vi "UHR-Fleezers Control (fpga) - 11.5_testing.vi"() -> ()   [LabVIEW 2012]
doc: "UHR-Fleezers Instrument Control Code (fpga)"
uses:
  Downloads/HandshakingLV2011/Handshaking/FPGAHandShakeState.ctl
  <vilib>/Platform/TimedLoop/XDataNode/timing_clust.ctl
  <vilib>/Platform/TimedLoop/XDataNode/nitl_modes.ctl
  <vilib>/Platform/TimedLoop/XDataNode/wakeup.ctl
  <vilib>/rvi/eio/common/nirviEmuTemplateMethod_errors.vi
  <vilib>/rvi/Emulation/niFpgaSctlEmulationGetInTimedLoop.vi
  <vilib>/rvi/DataTransferAndStorage/Container/Common/niFpgaContainerGetUniqueNameForEmu.vi
  <vilib>/rvi/FIFO/Fifo_Resource/nirvififoEmulationSetSize.vi
  <vilib>/rvi/Emulation/niFpgaSctlEmulationFifoFullMgr.vi
  <vilib>/rvi/errors/niFpgaSetErrorForExecOnDevCompSimple.vi
  <vilib>/rvi/eio/common/nirviEmuReportErrorAndStop.vi
  <vilib>/rvi/interface/RandomDataEmulation/nirviRandomDataFPGAFIFO.vi
  <vilib>/rvi/interface/RandomDataEmulation/niFpgaRandomDataHandleErrors.vi
  <vilib>/rvi/Emulation/niFpgaSctlEmulationGlobalWrite.vi
  <vilib>/rvi/Emulation/niFpgaSctlEmulationRegisterWithScheduler.vi
  <vilib>/rvi/Emulation/niFpgaSctlEmulationScheduler.vi
  <vilib>/rvi/DataTransferAndStorage/Container/Common/niFpgaContainerExecOnDevCompGetState.vi
  <vilib>/rvi/Memory/Memory_Emulation/niFpgaMemoryEmulationCacheClearOnFirstRun.vi
  <vilib>/rvi/Memory/Memory_Emulation/nirvimemoryEmulationManagerCache_MakeExclusive.vi
  <vilib>/rvi/Memory/Memory_Emulation/niFpgaMemoryEmulationValidateCache.vi
  <vilib>/rvi/Memory/Memory_Emulation/nirvimemoryEmulationManagerCache_ReleaseExclusive.vi
  <vilib>/rvi/Memory/Memory_Emulation/nirvimemoryEmulationManagerCache_InsertValue.vi
  <vilib>/Utility/error.llb/Clear Errors.vi
  <vilib>/rvi/Memory/Memory_Emulation/nirvimemoryEmulationManagerCache_GetValue.vi
  <vilib>/rvi/Memory/Memory_Emulation/nirvimemoryEmulationManagerCache_SetValue.vi
  <vilib>/rvi/Emulation/niFpgaSctlEmulationResourceMgr.vi
  <vilib>/Platform/TimedLoop/XDataNode/XDataNode.xnode
  <vilib>/eio/EIOMethodNode/EIOMethodNode.xnode
  <vilib>/eio/EIONode/EIONode.xnode
  <vilib>/rvi/DataTransferAndStorage/Container/XNode/niFpgaContainer.xnode
  <vilib>/rvi/FIFO/Fifo_Resource/nirvififoEmulationRead.vi
  <vilib>/rvi/interface/RandomDataEmulation/nirviRandomDataFpgaReadWriteTemplate.vi
  <vilib>/rvi/Memory/Memory_Emulation/niFpgaMemoryEmulationRefIn.vi
  <vilib>/rvi/FIFO/Fifo_Resource/nirvififoEmulationWrite.vi
  <vilib>/addons/control/pid/fpga.llb/XNode/niFpgaPID.xnode
  <vilib>/Platform/TimedLoop/XDataNode/XDNodeRunTimeDep.lvlib
panel:
  in  "N trap osc periods":i16
  in  "Trap osc period (pts)":i16
  in  "Initiate trap osc":bool
  in  "Osc trap 2":bool
  in  "Data":i32
  in  "Address 2":u32
  in  "Ready Write":bool
  in  "Tab Control":T1(tab)=enum."Force FB"
  in  "Set 3":bool
  in  "Set 2":bool=TRUE
  in  "Set 1":bool=TRUE
  in  "Trap Pos to FIFO":bool
  in  "N of AI1 Int Acq Sets":i16=2 min=1 max=3 step=1
  out "AI Late Counter":u8
  in  "ai count":u16=400
  in  "+ phase":bool
  in  "Phase count adjustment":i16
  out "Relative phase":i16
  in  "AI to FIFO":bool
  out "BD1 Frequency Out 1":u64
  out "BD1 Frequency Out 2":u64
  out "Trap Pos FIFO Timeout":u16
  out "Trap AI FIFO Timeout":u16
  in  "Trap FIFO Set Timeout":i32
  in  "Tab Control 2":T2(tab)
  in  "RD":bool
  in  "FB1 output high":i16=3000
  in  "FB1 output low":i16
  in  "D1":i16
  in  "I1":i16=5
  in  "P1":i16=10
  in  "Swap F1 and F2":bool
  in  "Cont. Scan":bool
  in  "Abort scan":bool
  in  "Cycles per step":u64
  in  "Scan BD":bool
  in  "Number of scans":u16
  in  "Scan steps":u64
  in  "Scan freq.  increment":i64
  out "Scanning":bool
  in  "Start scan":bool
  in  "OSK Bd 1":bool
  in  "Reset Bd 1":bool
  in  "PMODE":bool
  in  "Direct RF Box \nCommunication":bool
  in  "Data BD 2":u8 format="%08b"
  in  "Data BD 1":u8 format="%08b"
  in  "Address":u8 format="%02x"
  in  "Update Data":bool
  in  "FPGA Controls\n RF Box":bool
  in  "Number Interlace Cycles":u8=2 min=1 max=3
  in  "Interlace Off Parameters":u8=1 min=1 max=3
  in  "Interlace ON/OFF":bool
  out "DIO Relative phase":i16
  in  "Phase count adjustment (DIO)":i16
  in  "+ phase (DIO)":bool
  out "DIO Late Counter":u8
  in  "DIO count 1 (ticks)":u16=400
  in  "DIO count 2 (ticks)":u16=400
  in  "DIO count 3 (ticks)":u16=400
  out "AI2 Y Sum Set 2":i16
  out "AI2 Y Sum Set 1":i16
  in  "FB Setpoint Set 1":i16 min=0 step=1
  in  "FB Reset Set 1":bool
  in  "FB On/Off Set 1":bool
  in  "FB Reset Set 2":bool
  in  "FB On/Off Set 2":bool
  in  "FB Setpoint Set 2":i16 min=0 step=1
  out "Scan I":u64
  in  "Amp switch delay":u8=5
  in  "XY phase ext loop method":bool
  in  "BD 2 Amplitude 1":u16
  in  "BD 1 Amplitude 1":u16
  in  "BD 2 Frequency 1":u64
  in  "BD 1 Frequency 1":u64
  in  "BD 2 Amplitude 2":u16
  in  "BD 1 Amplitude 2":u16
  in  "BD 2 Frequency 2":u64
  in  "BD 1 Frequency 2":u64
  in  "BD 2 Amplitude 3":u16
  in  "BD 1 Amplitude 3":u16
  in  "BD 2 Frequency 3":u64
  in  "BD 1 Frequency 3":u64
  in  "BD 1 Delay (ticks)":u8
  in  "BD 2 Delay (Ticks)":u8 caption="Count(Ticks)"
  in  "Next trap write delay (ticks)":u8 caption="Count(Ticks)"
  in  "Amp switch delay 2":u8=5
  in  "BD 2 Delay (Ticks) 2":u8 caption="Count(Ticks)"
  in  "BD 1 Delay (ticks) 2":u8
  in  "FB2 output high":fxp<+/-,16,1>=0.999969482421875
  in  "FB2 output low":fxp<+/-,16,1>=-1.0
  in  "P2":fxp<+/-,16,8> format="%.11g"
  in  "I2":fxp<+/-,16,8>=10.0 format="%.11g"
  in  "D2":fxp<+/-,16,8> format="%.11g"
  in  "Negate Diff?":bool
  in  "Diff FB Measurement?":bool
  in  "FB Trig Integrate":u32=1
  out "TTrig?":bool
  in  "TTrig Negate Pos":bool=TRUE
  out "Trap Pos FB Int Signal":fxp<+/-,24,9> format="%.18g"
  out "Trap Pos FB Int-Norm Signal":fxp<+/-,16,1> format="%.16g"
  in  "FPGA TTrig Thresh":i64
  in  "FPGA Trap Trig":bool
  out "Trap Pos FB Action":i64
  in  "Trap Pos. FB Offset Factor":i64
  in  "Trap Pos. FB Mult Factor":i64=2
  in  "Trap Pos. FB Reset":bool
  in  "Trap Pos FB Monitor T1 or T2":bool
  in  "AI1 X Scale":u16
  in  "Trap Pos FB Int Count":u16=100
  in  "Trap Pos FB Negate Action":bool
  out "AI1 X Set 2":fxp<+/-,16,1>
  out "AI1 X Set 1":fxp<+/-,16,1>
  in  "Trap Pos. FB SP":fxp<+/-,16,1>
  in  "Force feedback":bool
  out "TTrig Sig":i64
  out "TTrig Fin Thresh":i64
  in  "1D or 2D Scan?":bool
  in  "Abort scan (MCL)":bool
  in  "MCL Scan Axis":bool
  in  "Cont. Scan (MCL)":bool
  out "Scan I (MCL)":u64
  in  "Number of scans (MCL)":u16
  out "Scanning MCL":bool
  in  "Scan steps (MCL)":u64
  in  "Cycles per step (MCL)":u64
  in  "Scan freq.  increment (MCL)":i16
  in  "Start scan (MCL)":bool
  in  "AO2":i16
  in  "AO1":i16
  out "MCL Late Counter":u8
  in  "MCL count":u32=800
  out "MCL Relative Phase":i16
  in  "Phase count adjustment (MCL)":i16
  in  "+ phase (MCL)":bool
  out "APD3 out state":bool
  in  "APD Gate Operating Mode":u8 max=2 step=1
  in  "Invert APD Gate":bool
  in  "APD Gate OFF Count":u16=100
  in  "APD Gate ON Count":u16=300
  out "APD 1 Gate Late Counter":u8
  out "APD 1 Gate Relative Phase":i16
  in  "Phase count adjustment (APD 1 Gate)":i16
  in  "+ phase (APD 1 Gate)":bool
  out "APD 2 Counts 0":u32
  out "APD 2 Counts 1":u32
  out "APD 1 Counts 0":u32
  out "APD 1 Counts 1":u32
  out "APD1 out state":bool
  in  "APD AO scale factor":i16=1
  in  "APD to FIFO":bool
  in  "APD Acq Rate Count":u32=20000000
  out "APD Acq Late Counter":u8
  out "APD Acq Relative Phase":i16
  in  "Phase Count Adjustment (APD Acq)":i16
  in  "+ phase (APD Acq)":bool
  in  "Phase count adjustment (APD 2 Gate)":i16
  out "APD 2 Gate Late Counter":u8
  out "APD 2 Gate Relative Phase":i16
  in  "+ phase (APD 2 Gate)":bool
  out "APD2 out state":bool
  out "APD 3 Counts 0":u32
  out "APD 3 Counts 1":u32
  out "APD 3 Gate Late Counter":u8
  in  "Phase count adjustment (APD 3 Gate)":i16
  out "APD 3 Gate Relative Phase":i16
  in  "+ phase (APD 3 Gate)":bool
  in  "D3":i16
  in  "I3":i16=5
  in  "P3":i16=10
  in  "Green Filter Flipper":bool
  in  "Green FB Count":u16=1200
  out "Green Late Counter":u8
  out "Green FB Relative Phase":i16
  in  "Phase count adjustment (Green FB)":i16=10
  in  "+ phase (Green FB)":bool
  out "Green FB Sum":i16
  in  "Green int current ON count adj":u16=150
  in  "Current Out":u16=30000
  in  "Green FB On/Off":bool
  in  "Green FB Setpoint":i16=250 min=0 step=1
  in  "Green FB Reset":bool
  in  "Operating Mode 2":u8=2 max=2 step=1
  in  "Invert GI 2":bool
  in  "Green interlace OFF count 2":u16=900
  in  "Green interlace ON count 2":u16=300
  out "GI Late Counter 2":u8
  out "GI Relative phase 2":i16
  in  "Phase count adjustment (GI) 2":i16=20
  in  "+ phase (GI) 2":bool
  in  "Green interlace OFF count":u16=100
  out "GI Relative phase":i16
  in  "Phase count adjustment (GI)":i16
  in  "+ phase (GI)":bool
  in  "Green interlace ON count":u16=300
  out "GI Late Counter":u8
  in  "Invert GI":bool
  in  "Operating Mode":u8 max=2 step=1
  in  "+ phase (RI)":bool
  out "RI Relative phase":i16
  out "RI Late Counter":u8
  in  "Red interlace ON count":u16=300
  in  "Red interlace OFF count":u16=100
  in  "Invert RI":bool
  in  "Red Laser Operating Mode":u8 max=2 step=1
  in  "Phase count adjustment (RI)":i16
  out "Red FB Intensity":i16
  in  "RI Current Out":u16=30000
  in  "Red FB On/Off":bool
  in  "D4":i16
  in  "I4":i16=5
  in  "P4":i16=10
  in  "Red FB Setpoint":i16=250 min=0 step=1
  in  "Red FB Reset":bool
  in  "RI Operating Mode 2":u8=2 max=2 step=1
  in  "Invert RI 2":bool
  in  "Phase count adjustment (BI AO)":i16=20
  in  "Blue current ON count adj (AO)":u16=150
  in  "BI Current Out":i16=30000
  in  "Blue FB On/Off":bool
  in  "D5":i16
  in  "I5":i16=5
  in  "P5":i16=10
  in  "Blue FB Setpoint":i16=250 min=0 step=1
  in  "Blue FB Reset":bool
  in  "BI Operating Mode (AO)":u8=2 max=2 step=1
  in  "Invert BI (AO)":bool
  in  "Blue OFF count (AO)":u16=900
  in  "Blue ON count (AO)":u16=300
  out "BI Late Counter (AO)":u8
  out "BI Relative phase (AO)":i16
  in  "+ phase (BI AO)":bool
  in  "Phase count adjustment (BI D)":i16
  in  "Blue Laser Operating Mode (D)":u8 max=2 step=1
  in  "Invert BI (D)":bool
  in  "Blue interlace OFF count (D)":u16=100
  in  "Blue interlace ON count (D)":u16=300
  out "Blue Late Counter (D)":u8
  out "BI Relative phase (D)":i16
  in  "+ phase (BI D)":bool
  out "Blue Intensity":i16
  # "Only one of these can be on\nat a time:"
  # "Raster Scan AOD"
  # "1 (X)"
  # "2 (Y)"
  # "IR Intensity Feedback (RF BD 1)"
  # "FB Gains Set 1"
  # "FB output range 1"
  # "False is usual, True is external loop method"
  # "Parameters if using the external RF switching loop"
  # "Parameters if using the usual internal RF switching method"
  # "FB Triggering Excitation Laser"
  # "Trap Pos. FB Gains"
  # "Trap Pos. FB Range"
  # "AO1 (Y)"
  # "2D"
  # "1D"
  # "AO2 (X)"
  # "APD AO for aligning"
  # "Detection Loop"
  # "Green fluorescent laser digital gate interlacing loop"
  # "0 Forced ON\n1 Forced OFF\n2 Interlacing"
  # "Green FB Gains"
  # "Red fluorescent laser digital gate interlacing loop"
  # "Detection Loop"
  # "0 Forced ON\n1 Forced OFF\n2 Interlacing"
  # "Analog/FB Control Loop\n(Disabled)"
  # "Digital Control Loop"
  # "Blue laser intensity reading"
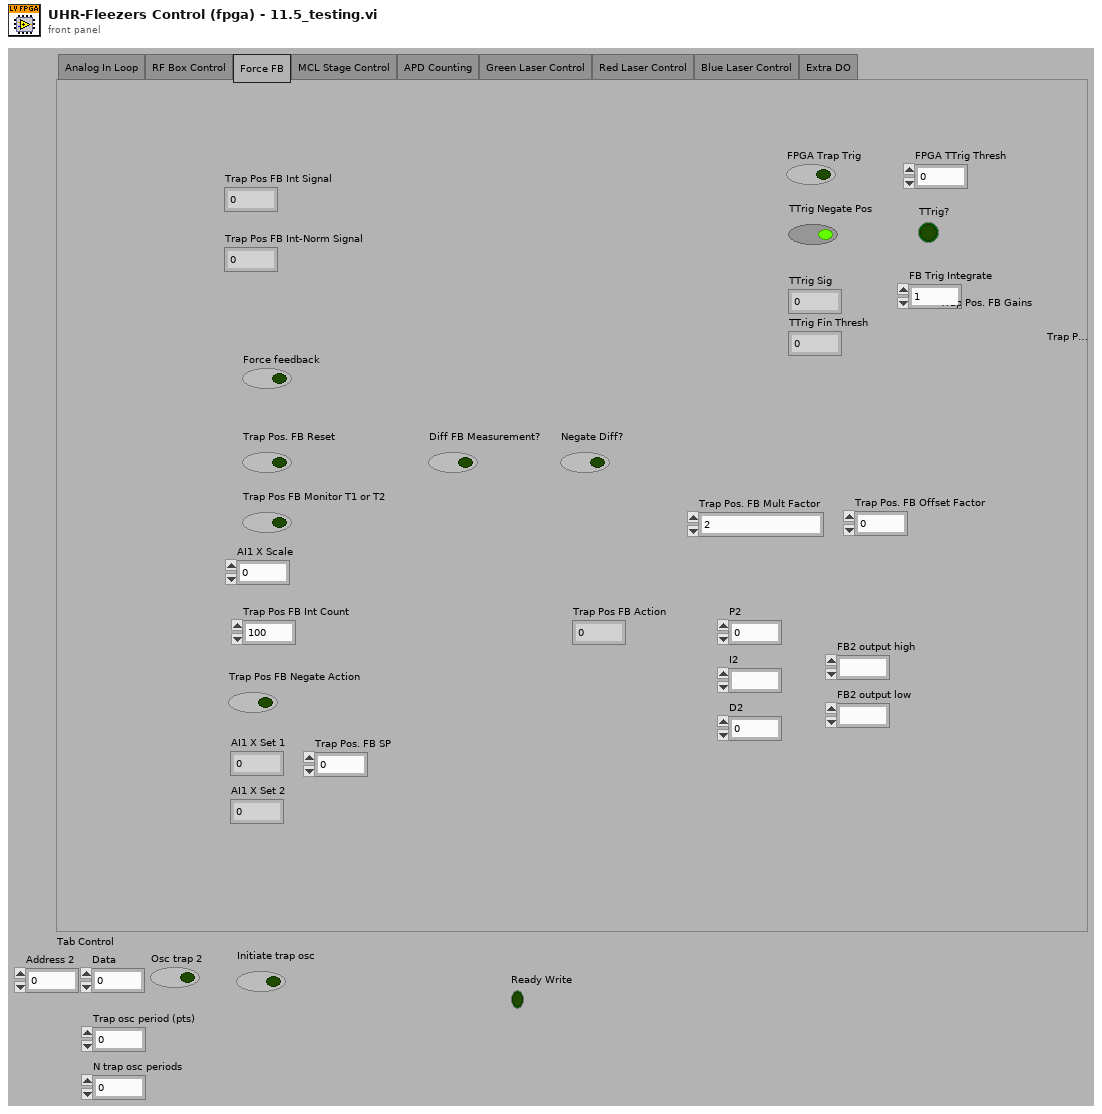
[diagram p1: front panel]
types:
  T1 = enum32{"Analog In Loop", "RF Box Control", "Force FB", "MCL Stage Control", "APD Counting", "Green Laser Control", "Red Laser Control", "Blue Laser Control", "Extra DO"}
  T2 = enum32{"Controls", "Interlacing Frequency and Amplitude Values"}
  T3 = typedef "FPGAHandShakeState.ctl" = enum16{"Wait Ready", "ReadWrite", "UnSet Ready"}
  T4 = typedef "XDNodeRunTimeDep.lvlib/timing_clust.ctl" = cluster{"Expected End [f-1]":u64, "Actual End [f-1]":u64, "Finished Late? [f-1]":bool, "Expected End [i-1]":u64, "Actual End [i-1]":u64, "Finished Late? [i-1]":bool, "Expected Start [i]":u64, "Actual Start [i]":u64, "Expected Start [f]":u64, "Actual Start [f]":u64, "Source Name":string, "Structure Name":string, "Period":i64, "Deadline":i64, "Offset":i64, "Start":i64, "Priority":i32, "Timeout":i32, "Mode":T5, "Wakeup Reason":T6, "Error":errorcluster, "Source Type":string, "Secondary Source Type":string, "Global End Time":u64, "Global Start Time":u64, "Frame Duration":u64, "Iteration Duration":u64, "Assigned CPU":i32, "I/O Scan Engine Mode":u32}
  T5 = typedef "XDNodeRunTimeDep.lvlib/nitl_modes.ctl" = enum32{"No Change", "Process missed periods, maintain original phase", "Discard missed periods, maintain original phase", "Process missed periods, ignore original phase", "Discard missed periods, ignore original phase"}
  T6 = typedef "XDNodeRunTimeDep.lvlib/wakeup.ctl" = enum32{"Normal", "Aborted", "Asynchronous wakeup", "Timing source error", "Timed loop error", "Timeout"}
  T7 = cluster{"proportional gain (Kc)":i16, "integral gain (Kc*Ts/Ti)":i16, "derivative gain (Kc*Td/Ts)":i16}
  T8 = cluster{"FB1 output high":i16, "FB1 output low":i16}
  T9 = cluster{"P2":fxp<+/-,16,8>, "I2":fxp<+/-,16,8>, "D2":fxp<+/-,16,8>}
  T10 = cluster{"FB2 output high":fxp<+/-,16,1>, "FB2 output low":fxp<+/-,16,1>}
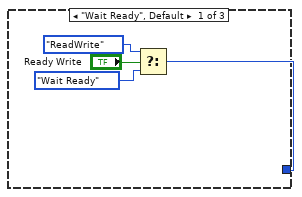
[diagram p2: hidden frame]
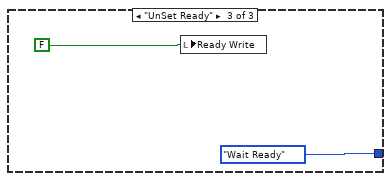
[diagram p3: hidden frame]
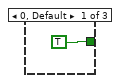
[diagram p5: hidden frame]
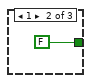
[diagram p6: hidden frame]
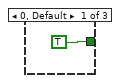
[diagram p7: hidden frame]
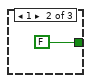
[diagram p8: hidden frame]
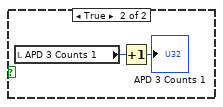
[diagram p9: hidden frame]
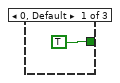
[diagram p10: hidden frame]
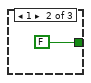
[diagram p11: hidden frame]
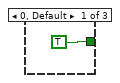
[diagram p12: hidden frame]
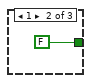
[diagram p13: hidden frame]
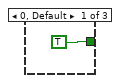
[diagram p14: hidden frame]
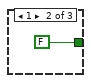
[diagram p15: hidden frame]
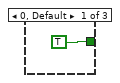
[diagram p16: hidden frame]
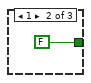
[diagram p17: hidden frame]
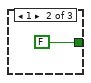
[diagram p20: hidden frame]
diagram:
  w4 = u16 0
  w6 = FALSE
  w3 = FALSE
  # "timing array current index"
  # "timing array"
  # "timing counter (phase adjusted here)"
  # "late counter"
  n1 = while "External XY RF switching timing loop" {
    stop <- FALSE stop-if-true
    # "This loop is stalled until the RF FIFO get a value, which only happens if we are using the external loop RF switching method. With this method we gain additional delay time (because \nwe allow the rest of the main RF loop to procede while this loop waits to send the switch signals - a form of parallelism). Probably this is always the method to use. Helps to simplify \nthe main RF code. If it works reliably, could take out the redundant code in the main RF loop to save space and simplify."
    n2 = xnode "FIFO Read"("Timeout"=-1) -> ("Element"=w16:bool)  [unwired: 1 in, 2 out]
    n3 = flat-sequence "BD 1 (X)" {
      tunnel: w16 -> [w25]
      tunnel: [w25] -> w15
      tunnel: w15 -> [w27]
      tunnel: "Amp switch delay 2" -> [w28]
      frame #0 {
        n4 = call "Wait9"("Count(Ticks)"="BD 1 Delay (ticks) 2") -> ()  [unwired: 1 out]
      }
      frame #1 {
        # "switch frequency"
        n5 = xnode "FPGA I/O Node"("Connector1/DIO36"=w27) -> ()  [unwired: 1 in, 1 out]
      }
      frame #2 {
        # "~5 ticks is usual"
        n6 = call "Wait10"("Count(Ticks)"=w28) -> ()  [unwired: 1 out]
      }
      frame #3 {
        # "this switches amplitude"
        # "switch amplitude"
        # "send udclk high"
        n7 = xnode "FPGA I/O Node"("Connector1/DIO30"=TRUE ("Connector1/DIO15")) -> ()  [unwired: 1 in, 1 out]
      }
      frame #4 {
        # "reset to be ready for next\ncycle"
        # "send udclk low"
        n8 = xnode "FPGA I/O Node"("Connector1/DIO30"=FALSE ("Connector1/DIO15")) -> ()  [unwired: 1 in, 1 out]
      }
    }
    n9 = flat-sequence "BD 2 (Y)" {
      tunnel: w16 -> [w19]
      tunnel: [w19] -> w14
      tunnel: w14 -> [w21]
      tunnel: "Amp switch delay 2" -> [w22]
      frame #0 {
        n10 = call "Wait11"("Count(Ticks)"="BD 2 Delay (Ticks) 2") -> ()  [unwired: 1 out]
      }
      frame #1 {
        # "switch frequency"
        n11 = xnode "FPGA I/O Node"("Connector1/DIO37"=w21) -> ()  [unwired: 1 in, 1 out]
      }
      frame #2 {
        # "~5 ticks is usual"
        n12 = call "Wait12"("Count(Ticks)"=w22) -> ()  [unwired: 1 out]
      }
      frame #3 {
        # "this switches amplitude"
        # "switch amplitude"
        # "send udclk high"
        n13 = xnode "FPGA I/O Node"("Connector1/DIO29"=TRUE ("Connector1/DIO15")) -> ()  [unwired: 1 in, 1 out]
      }
      frame #4 {
        # "reset to be ready for next\ncycle"
        # "send udclk low"
        n14 = xnode "FPGA I/O Node"("Connector1/DIO29"=FALSE ("Connector1/DIO15")) -> ()  [unwired: 1 in, 1 out]
      }
    }
  }
  n15 = flat-sequence "FPGA initialization to do before running any of the loops" {
    tunnel: [u16 0 ("DIO count 3 (ticks)")] -> w2
    tunnel: [w32] -> _
    frame #0 {
      w31 = FALSE ("Enable")
      # "BD 2 (Y)"
      # "BD 1 (X)"
      # "Start up expansion chassis early\nto avoid delays later"
      # "This pin controls udclk on the RF boards.\nWhen initially configuring the boards, this pin needs to be\nconfigured as a high impedance input.  Later it will be switched\nto an output."
      # "Initial setting of DIO data and \naddress to low (before reset).  \nThis needs to happen before the other\ncontrol method loops execute."
      n16 = xnode "FPGA I/O Node"("Chassis2/Mod4/AO0"=u16 0) -> ("Chassis2/Mod1/AI0"=w32:i16)  [unwired: 2 in, 2 out]
      n17 = xnode "FPGA I/O Method Node"("Enable"=w31) -> ()  [unwired: 1 in, 1 out]
      n18 = xnode "FPGA I/O Method Node"("Enable"=w31) -> ()  [unwired: 1 in, 1 out]
      n19 = xnode "FPGA I/O Node"("Connector1/DIO0"=FALSE, "Connector1/DIO1"=FALSE, "Connector1/DIO2"=FALSE, "Connector1/DIO3"=FALSE, "Connector1/DIO4"=FALSE, "Connector1/DIO5"=FALSE, "Connector1/DIO6"=FALSE, "Connector1/DIO7"=FALSE, "Connector1/DIO8"=FALSE, "Connector1/DIO9"=FALSE, "Connector1/DIO10"=FALSE, "Connector1/DIO11"=FALSE, "Connector1/DIO12"=FALSE, "Connector1/DIO13"=FALSE, "Connector1/DIO15"=FALSE, "Connector1/DIO20"=FALSE, "Connector1/DIO21"=FALSE, "Connector1/DIO22"=FALSE, "Connector1/DIO23"=FALSE, "Connector1/DIO24"=FALSE, "Connector1/DIO25"=FALSE, "Connector1/DIO26"=FALSE, "Connector1/DIO27"=FALSE, "Connector1/DIO14"=FALSE) -> ()  [unwired: 24 in, 24 out]
    }
  }
  n20 = local read "AO1"() -> (w11:i16)
  n21 = local read "AO2"() -> (w10:i16)
  n22 = node-c288() -> (w9:T4)  [unwired: 1 in]
  n23 = timed-loop "RF box board DIO control: control bits" {
    timing: w9 -> [_]
    timing-out: [_] -> w8
    tunnel: [w61] -> _
    tunnel: w2 -> [w61]
    stop <- FALSE stop-if-true
    n24 = xnode "FPGA I/O Node"("Connector1/DIO16"="RD", "Connector1/DIO17"="PMODE", "Connector1/DIO18"="OSK Bd 1", "Connector1/DIO19"="Reset Bd 1", "Connector0/DIO3"="Green Filter Flipper") -> ()  [unwired: 5 in, 5 out]
  }
  n25 = while "RF box board DIO control: parallel communication" {
    shift-right: [w74] -> _
    shift-left: w2 -> [w73]
    shift-right: [w72] -> _
    shift-left: FALSE ("Swap F1 and F2") -> [w71]
    stop <- FALSE stop-if-true
    n26 = flat-sequence {
      tunnel: w71 -> [w78]
      tunnel: w73 -> [w76]
      tunnel: [w78] -> w70
      tunnel: [w77] -> w69
      tunnel: [w76] -> w68
      tunnel: [w84] -> w74
      tunnel: [w83] -> w72
      tunnel: w70 -> [w82]
      tunnel: w69 -> [w80]
      tunnel: w68 -> [w79]
      frame #0 {
        n27 = call "Loop Timer"("Count(Ticks)"=w76) -> ("Tick Count(Ticks)"=w77:u16)
      }
      frame #1 {
        n28 = flat-sequence {
          tunnel: ["FPGA Controls\n RF Box"] -> w81
          tunnel: w82 -> [w85]
          tunnel: [w139] -> w84
          tunnel: [w152] -> w83
          tunnel: w81 -> [w151]
          tunnel: w80 -> [w145]
          tunnel: w79 -> [w142]
          frame #0 {
            n29 = case shown="True" "FPGA Controls\n RF Box" {
              tunnel: w85 -> [_ w87]
              frame False {
              }
              frame True {
                n30 = flat-sequence {
                  tunnel: w87 -> [w97]
                  frame #0 {
                    n31 = First Call?() -> (First Call?: T/F=w88:bool)
                    n32 = case shown="True" w88 {
                      frame False {
                      }
                      frame True {
                        # "BD 2"
                        # "BD 1"
                        # "If first time data updated, be sure to set WR high and UDCLK low\nbefore setting data and address bits."
                        n33 = xnode "FPGA I/O Method Node"("Enable"=TRUE) -> ("FPGA I/O Out"=w90:refnum<k21>)  [unwired: 1 in]
                        n34 = xnode "FPGA I/O Method Node"("Enable"=TRUE) -> ("FPGA I/O Out"=w93:refnum<k21>)  [unwired: 1 in]
                        n35 = xnode "FPGA I/O Node"("Connector1/DIO15"=TRUE) -> ()  [unwired: 1 in, 1 out]
                        n36 = xnode "FPGA I/O Node"("I/O Item"=FALSE ("Connector1/DIO30"), "FPGA I/O In"=w90) -> ()  [unwired: 1 out]
                        n37 = xnode "FPGA I/O Node"("I/O Item"=FALSE ("Connector1/DIO30"), "FPGA I/O In"=w93) -> ()  [unwired: 1 out]
                      }
                    }
                  }
                  frame #1 {
                    n38 = case shown="True" "XY phase ext loop method" {
                      tunnel: w97 -> [w99 w111]
                      frame False {
                        # "Usual operation"
                        n39 = flat-sequence "BD 1 (X)" {
                          tunnel: w99 -> [w106]
                          tunnel: "Amp switch delay" -> [w107]
                          frame #0 {
                            n40 = call "Wait6"("Count(Ticks)"="BD 1 Delay (ticks)") -> ()  [unwired: 1 out]
                          }
                          frame #1 {
                            # "switch frequency"
                            n41 = xnode "FPGA I/O Node"("Connector1/DIO36"=w106) -> ()  [unwired: 1 in, 1 out]
                          }
                          frame #2 {
                            # "~5 ticks is usual"
                            n42 = call "Wait4"("Count(Ticks)"=w107) -> ()  [unwired: 1 out]
                          }
                          frame #3 {
                            # "this switches amplitude"
                            # "switch amplitude"
                            # "send udclk high"
                            n43 = xnode "FPGA I/O Node"("Connector1/DIO30"=TRUE ("Connector1/DIO15")) -> ()  [unwired: 1 in, 1 out]
                          }
                          frame #4 {
                            # "reset to be ready for next\ncycle"
                            # "send udclk low"
                            n44 = xnode "FPGA I/O Node"("Connector1/DIO30"=FALSE ("Connector1/DIO15")) -> ()  [unwired: 1 in, 1 out]
                          }
                        }
                        n45 = flat-sequence "BD 2 (Y)" {
                          tunnel: w99 -> [w101]
                          tunnel: "Amp switch delay" -> [w102]
                          frame #0 {
                            n46 = call "Wait7"("Count(Ticks)"="BD 2 Delay (Ticks)") -> ()  [unwired: 1 out]
                          }
                          frame #1 {
                            # "switch frequency"
                            n47 = xnode "FPGA I/O Node"("Connector1/DIO37"=w101) -> ()  [unwired: 1 in, 1 out]
                          }
                          frame #2 {
                            # "~5 ticks is usual"
                            n48 = call "Wait5"("Count(Ticks)"=w102) -> ()  [unwired: 1 out]
                          }
                          frame #3 {
                            # "this switches amplitude"
                            # "switch amplitude"
                            # "send udclk high"
                            n49 = xnode "FPGA I/O Node"("Connector1/DIO29"=TRUE ("Connector1/DIO15")) -> ()  [unwired: 1 in, 1 out]
                          }
                          frame #4 {
                            # "reset to be ready for next\ncycle"
                            # "send udclk low"
                            n50 = xnode "FPGA I/O Node"("Connector1/DIO29"=FALSE ("Connector1/DIO15")) -> ()  [unwired: 1 in, 1 out]
                          }
                        }
                      }
                      frame True {
                        # "Operation when you need a long delay for either X or Y to synchonize AOD light out phase (> ~100 ticks)."
                        # "Trigger the external loop by sending the boolean FSK value through a FIFO"
                        n51 = xnode "FIFO Write"("Element"=w111, "Timeout"=-1) -> ()  [unwired: 1 in, 2 out]
                      }
                    }
                  }
                }
              }
            }
          }
          frame #1 {
            # "This is the prior cycle's on time"
            # "increment timing\nindex, reset to 0 if \nend of matrix"
            # "Reset to begginning (1) when number of cycles reached."
            # "timing index"
            # "build byte stacks for writing data\n(must correspond to addresses array constant)"
            # "Timing housekeeping"
            # "Adjust phase if late\n(maintains constant phase relationship between cycles)"
            n52 = Bundle("FB1 output high"="FB1 output high", "FB1 output low"="FB1 output low") -> (w112:T8)  [unwired: 1 in]
            n53 = Bundle("P1"="P1", "I1"="I1", "D1"="D1") -> (w113:cluster{"P1":i16, "I1":i16, "D1":i16})  [unwired: 1 in]
            n54 = feedback #1(u8 0 ("t")) -> (w148:u8)
            n55 = Increment(x=w148) -> (x+1=w192:u8)
            n56 = Increment(x="Number Interlace Cycles") -> (x+1=w187:u8)
            n57 = Equal?(x=w192, y=w187) -> (x = y?=w194:bool)
            n58 = Select(t=u8 1, s=w194, f=w192) -> (s? t:f=w147:u8)
            n59 = feedback-in #1(w147) -> ()
            n60 = Increment(x=w147) -> (x+1=w189:u8)
            n61 = Equal?(x=w189, y=w187) -> (x = y?=w190:bool)
            n62 = Select(t=u8 1, s=w190, f=w189) -> (s? t:f=w186:u8)
            n63 = Select(t=w186, s="Interlace ON/OFF", f="Interlace Off Parameters") -> (s? t:f=w170:u8)
            n64 = case shown="2" w170 {
              tunnel: [w271 "BD 1 Frequency 2" "BD 1 Frequency 3"] -> w182
              tunnel: [w270 "BD 2 Frequency 2" "BD 2 Frequency 3"] -> w171
              tunnel: ["BD 2 Amplitude 1" "BD 2 Amplitude 2" "BD 2 Amplitude 3"] -> w127
              tunnel: [w259 w435 "BD 1 Amplitude 3"] -> w130
              tunnel: w113 -> [w233 w432 _]
              tunnel: w112 -> [w234 w431 _]
              frame 1, Default {
                w250 = fxp<+/-,24,9> 0.0 ("AI1 X Set 2")
                w243 = u16 0
                w266 = u64 0 ("f")
                # "This signal integration happens no matter what\nso that correct setpoints can be chosen before \nturning on the FB."
                # "Trap 1"
                n65 = local read "AI1 X Set 2"() -> (w246:fxp<+/-,16,1>)
                n66 = local read "AI1 X Set 1"() -> (w247:fxp<+/-,16,1>)
                n67 = local read "Scanning"() -> (w272:bool)
                n68 = Or(x=w272, y="Start scan") -> (x .or. y?=w264:bool)
                n69 = case shown="False" "Diff FB Measurement?" {
                  tunnel: w246 -> [w280 w289]
                  tunnel: w247 -> [w279 w290]
                  tunnel: [w277 w281] -> w248
                  frame False {
                    n70 = Select(t=w279, s="Trap Pos FB Monitor T1 or T2", f=w280) -> (s? t:f=w277:fxp<+/-,16,1>)
                  }
                  frame True {
                    n71 = Subtract(x=w290, y=w289) -> (x-y=w282:fxp<+/-,17,2>)
                    n72 = Not(x="Negate Diff?") -> (.not. x?=w288:bool)
                    n73 = Boolean To (0,1)(Boolean="Negate Diff?") -> (0, 1=w286:i16)
                    n74 = Boolean To (0,1)(Boolean=w288) -> (0, 1=w287:i16)
                    n75 = Negate(x=w286) -> (-x=w285:i16)
                    n76 = Add(x=w285, y=w287) -> (x+y=w283:i16)
                    n77 = Multiply(x=w283, y=w282) -> (x*y=w281:fxp<+/-,32,17>)
                  }
                }
                n78 = Not(x="Abort scan") -> (.not. x?=w262:bool)
                n79 = And(x=w262, y=w264) -> (x .and. y?=w261:bool)
                n80 = case "For raster scanning" shown="True" w261 {
                  tunnel: [u64 0 w416] -> w267
                  tunnel: "Start scan" -> [_ w401]
                  frame False {
                    n81 = local write "Scanning"(FALSE ("scanning")) -> ()
                  }
                  frame True {
                    w385 = i64 0
                    w384 = u64 0
                    # "scan incr."
                    # "freq. incr. mult."
                    # "count steps"
                    # "count number of cycles"
                    n82 = feedback #2(w384) -> (w413:u64)
                    n83 = Select(t=w384, s=w401, f=w413) -> (s? t:f=w415:u64)
                    n84 = Increment(x=w415) -> (x+1=w412:u64)
                    n85 = Greater?(x="Cycles per step", y=w412) -> (0:w394:bool)
                    n86 = Select(t=w412, s=w394, f=w384) -> (s? t:f=w411:u64)
                    n87 = feedback-in #2(w411) -> ()
                    n88 = feedback #3(w384) -> (w410:u64)
                    n89 = Select(t=w384, s=w401, f=w410) -> (s? t:f=w405:u64)
                    n90 = Increment(x=w405) -> (x+1=w409:u64)
                    n91 = Add(x="Scan steps", y="Scan steps") -> (x+y=w408:u64)
                    n92 = Select(t=w405, s=w394, f=w409) -> (s? t:f=w389:u64)
                    n93 = Greater?(x=w408, y=w389) -> (0:w388:bool)
                    n94 = Select(t=w389, s=w388, f=w384) -> (s? t:f=w406:u64)
                    n95 = feedback-in #3(w406) -> ()
                    n96 = Equal?(x="Scan steps", y=w389) -> (x = y?=w393:bool)
                    n97 = Greater?(x="Scan steps", y=w405) -> (0:w404:bool)
                    n98 = feedback #4(w385) -> (w407:i64)
                    n99 = Select(t=w385, s=w401, f=w407) -> (s? t:f=w391:i64)
                    n100 = Increment(x=w391) -> (x+1=w403:i64)
                    n101 = Decrement(x=w391) -> (x-1=w402:i64)
                    n102 = Select(t=w403, s=w404, f=w402) -> (s? t:f=w392:i64)
                    n103 = Select(t=w391, s=w393, f=w392) -> (s? t:f=w390:i64)
                    n104 = Select(t=w391, s=w394, f=w390) -> (s? t:f=w386:i64)
                    n105 = Select(t=w386, s=w388, f=w385) -> (s? t:f=w387:i64)
                    n106 = feedback-in #4(w387) -> ()
                    n107 = feedback #5(w384) -> (w400:u64)
                    n108 = Select(t=w384, s=w401, f=w400) -> (s? t:f=w396:u64)
                    n109 = Increment(x=w396) -> (x+1=w397:u64)
                    n110 = Select(t=w396, s=w388, f=w397) -> (s? t:f=w395:u64)
                    n111 = Greater?(x="Number of scans", y=w395) -> (0:w381:bool)
                    n112 = Multiply(x="Scan freq.  increment", y=w391) -> (x*y=w416:i64)
                    n113 = Select(t=TRUE, s="Cont. Scan", f=w381) -> (s? t:f=w380:bool)
                    "Scanning" <- w380
                    n114 = Select(t=w395, s=w380, f=w384) -> (s? t:f=w398:u64)
                    n115 = feedback-in #5(w398) -> ()
                    n116 = Increment(x=w395) -> (x+1=→"Scan I":u64)
                  }
                }
                n117 = feedback #6(w243) -> (w242:u16)
                n118 = Increment(x=w242) -> (x+1=w244:u16)
                n119 = Greater Or Equal?(x=w244, y="Trap Pos FB Int Count") -> (x >= y?=w235:bool)
                n120 = Select(t=w243, s=w235, f=w244) -> (s? t:f=w245:u16)
                n121 = feedback-in #6(w245) -> ()
                n122 = feedback #7(w250) -> (w249:fxp<+/-,24,9>)
                n123 = Add(x=w248, y=w249) -> (x+y=w241:fxp<+/-,24,9>)
                n124 = case "For intensity feedback" shown="True" "FB On/Off Set 1" {
                  tunnel: "BD 1 Amplitude 1" -> [w418 _]
                  tunnel: [w418 w422] -> w259
                  tunnel: w234 -> [_ w419]
                  tunnel: w233 -> [_ w420]
                  frame False {
                  }
                  frame True {
                    n125 = local read "AI2 Y Sum Set 1"() -> (w423:i16)
                    n126 = call "Slower PID.vi"("process variable"=w423, "reset?"="FB Reset Set 1", "setpoint"="FB Setpoint Set 1", "PID gains (x 2^8)"=w420, "output range"=w419) -> ("output"=w424:i16)  [unwired: 10 out]
                    n127 = To Unsigned Word Integer(number=w424) -> (unsigned 16bit integer=w422:u16)
                  }
                }
                n128 = Select(t=w250, s=w235, f=w241) -> (s? t:f=w253:fxp<+/-,24,9>)
                n129 = feedback-in #7(w253) -> ()
                n130 = Divide(x=w241, y="Trap Pos FB Int Count") -> (x/y=w236:fxp<+/-,16,1>)
                n131 = feedback #8(fxp<+/-,24,9> 0.0 ("AI1 X Set 2")) -> (w254:fxp<+/-,24,9>)
                n132 = Select(t=w241, s=w235, f=w254) -> (s? t:f=w255:fxp<+/-,24,9>)
                "Trap Pos FB Int Signal" <- w255
                n133 = feedback-in #8(w255) -> ()
                n134 = feedback #9(fxp<+/-,16,1> 0.0 ("Trap Pos FB Int-Norm Signal")) -> (w238:fxp<+/-,16,1>)
                n135 = Select(t=w236, s=w235, f=w238) -> (s? t:f=w237:fxp<+/-,16,1>)
                "Trap Pos FB Int-Norm Signal" <- w237
                n136 = feedback-in #9(w237) -> ()
                n137 = case "For position feedback" shown="True" "Force feedback" {
                  tunnel: [i64 0 w296] -> w256
                  tunnel: w236 -> [_ w293]
                  tunnel: w235 -> [_ w292]
                  frame False {
                  }
                  frame True {
                    n138 = feedback #10(i64 0) -> (w295:i64)
                    n139 = case shown="True" w292 {
                      tunnel: [w297 w311] -> w296
                      tunnel: w295 -> [w297 _]
                      tunnel: w293 -> [_ w305]
                      frame False {
                      }
                      frame True {
                        w315 = u32 0
                        n140 = Bundle("P2"="P2", "I2"="I2", "D2"="D2") -> (w301:T9)  [unwired: 1 in]
                        n141 = Bundle("FB2 output high"="FB2 output high", "FB2 output low"="FB2 output low") -> (w298:T10)  [unwired: 1 in]
                        n142 = xnode ("PID")("process variable"=w305, "reset?"="Trap Pos. FB Reset", "setpoint"="Trap Pos. FB SP", "PID gains"=w301, "output range"=w298) -> ("output"=w327:fxp<+/-,16,1>)
                        n143 = Negate(x=w327) -> (-x=w326:fxp<+/-,17,2>)
                        n144 = Select(t=w326, s="Trap Pos FB Negate Action", f=w327) -> (s? t:f=w323:fxp<+/-,17,2>)
                        n145 = Scale By Power Of 2(n=u32 15, x=u32 1) -> (x*2^n=w320:u32)
                        n146 = Multiply(x=w323, y=w320) -> (x*y=w319:fxp<+/-,17,17>)
                        n147 = To Quad Integer(1:w319) -> (0:w331:i64)
                        "Trap Pos FB Action" <- w331
                        n148 = Multiply(x=w331, y="Trap Pos. FB Mult Factor") -> (x*y=w329:i64)
                        n149 = Add(x=w329, y="Trap Pos. FB Offset Factor") -> (x+y=w311:i64)
                        n150 = feedback #11() -> (w312:i64)  [unwired: 1 in]
                        n151 = Add(x=w311, y=w312) -> (x+y=w309:i64)
                        n152 = feedback #12(w315) -> (w317:u32)
                        n153 = Increment(x=w317) -> (x+1=w306:u32)
                        n154 = Greater Or Equal?(x=w306, y="FB Trig Integrate") -> (x >= y?=w307:bool)
                        n155 = Select(t=i64 0, s=w307, f=w309) -> (s? t:f=w313:i64)
                        n156 = feedback-in #11(w313) -> ()
                        n157 = Select(t=w315, s=w307, f=w306) -> (s? t:f=w316:u32)
                        n158 = feedback-in #12(w316) -> ()
                        n159 = And(x=w307, y="FPGA Trap Trig") -> (x .and. y?=w314:bool)
                        n160 = case "Trap FB trigger excitation laser ON" shown="True" w314 {
                          tunnel: w309 -> [_ w335]
                          tunnel: w306 -> [_ w333]
                          frame False {
                          }
                          frame True {
                            n161 = Not(x="TTrig Negate Pos") -> (.not. x?=w342:bool)
                            n162 = Boolean To (0,1)(Boolean="TTrig Negate Pos") -> (0, 1=w340:i16)
                            n163 = Boolean To (0,1)(Boolean=w342) -> (0, 1=w341:i16)
                            n164 = Negate(x=w340) -> (-x=w339:i16)
                            n165 = Add(x=w339, y=w341) -> (x+y=w338:i16)
                            n166 = Multiply(x=w338, y=w335) -> (x*y=w337:i64)
                            "TTrig Sig" <- w337
                            n167 = Multiply(x="FPGA TTrig Thresh", y=w333) -> (x*y=w334:i64)
                            "TTrig Fin Thresh" <- w334
                            n168 = Greater Or Equal?(x=w337, y=w334) -> (x >= y?=w336:bool)
                            n169 = case shown="True" w336 {
                              frame False {
                              }
                              frame True {
                                w345 = TRUE ("Green FB On/Off")
                                w347 = u8 2 ("Operating Mode")
                                n170 = local write "Operating Mode 2"(w347) -> ()
                                n171 = local write "Operating Mode"(w347) -> ()
                                n172 = local write "Green FB On/Off"(w345) -> ()
                                n173 = local write "FPGA Trap Trig"(FALSE ("FPGA Trap Trig")) -> ()
                                "TTrig?" <- w345
                              }
                            }
                          }
                        }
                      }
                    }
                    n174 = feedback-in #10(w296) -> ()
                  }
                }
                n175 = Select(t=w266, s="Scan BD", f=w267) -> (s? t:f=w265:u64)
                n176 = Select(t=w267, s="Scan BD", f=w266) -> (s? t:f=w268:u64)
                n177 = Add(x=w265, y="BD 2 Frequency 1") -> (x+y=w270:u64)
                n178 = Compound Arithmetic op=ADD("BD 1 Frequency 1", w256, w268) -> (w271:u64)
                "BD1 Frequency Out 1" <- w271
              }
              frame 2 {
                # "Trap 2"
                n179 = case shown="True" "FB On/Off Set 2" {
                  tunnel: [w463 w466] -> w435
                  tunnel: "BD 1 Amplitude 2" -> [w463 _]
                  tunnel: w432 -> [_ w465]
                  tunnel: w431 -> [_ w464]
                  frame False {
                  }
                  frame True {
                    n180 = local read "AI2 Y Sum Set 2"() -> (w469:i16)
                    n181 = call "Slower PID.vi"("process variable"=w469, "reset?"="FB Reset Set 2", "setpoint"="FB Setpoint Set 2", "PID gains (x 2^8)"=w465, "output range"=w464) -> ("output"=w467:i16)  [unwired: 10 out]
                    n182 = To Unsigned Word Integer(number=w467) -> (unsigned 16bit integer=w466:u16)
                  }
                }
                n183 = Or(x="Osc trap 2", y="Initiate trap osc") -> (x .or. y?=w427:bool)
                n184 = case shown="True" w427 {
                  tunnel: [u64 0 ("y") w451] -> w429
                  tunnel: "Initiate trap osc" -> [_ w440]
                  frame False {
                  }
                  frame True {
                    w444 = u16 0
                    w442 = -1
                    n185 = local write "Initiate trap osc"(FALSE ("Initiate trap osc")) -> ()
                    n186 = feedback #13(w444) -> (w446:u16)
                    n187 = Select(t=w444, s=w440, f=w446) -> (s? t:f=w445:u16)
                    n188 = Greater Or Equal?(x=w445, y="Trap osc period (pts)") -> (x >= y?=w456:bool)
                    n189 = Or(x=w440, y=w456) -> (x .or. y?=w457:bool)
                    n190 = Select(t=u16 0, s=w457, f=w445) -> (s? t:f=w455:u16)
                    n191 = feedback #14(w442) -> (w443:i32)
                    n192 = Select(t=w442, s=w440, f=w443) -> (s? t:f=w441:i32)
                    n193 = Increment(x=w441) -> (x+1=w452:i32)
                    n194 = Equal?(x=w455, y=u16 0) -> (x = y?=w453:bool)
                    n195 = Increment(x=w455) -> (x+1=w461:u16)
                    n196 = feedback-in #13(w461) -> ()
                    n197 = xnode "Memory Read"("Address"=w455, "Memory In"=refnum<k21> "Trap osc memory") -> ("Data"=w451:i32)  [unwired: 1 out]
                    n198 = Select(t=w452, s=w453, f=w441) -> (s? t:f=w450:i32)
                    n199 = feedback-in #14(w450) -> ()
                    n200 = Greater Or Equal?(x=w450, y="N trap osc periods") -> (x >= y?=w448:bool)
                    n201 = Not(x=w448) -> (.not. x?=w447:bool)
                    n202 = local write "Osc trap 2"(w447) -> ()
                  }
                }
                n203 = Add(x="BD 1 Frequency 2", y=w429) -> (x+y=→"BD1 Frequency Out 2":u64)
              }
              frame 3 {
                # "Fluorescence period"
              }
            }
            n204 = feedback-in #15(w145) -> ()
            n205 = feedback #15(w145) -> (w144:u16)
            n206 = Select(t=w147, s="Interlace ON/OFF", f="Interlace Off Parameters") -> (s? t:f=w185:u8)
            n207 = Subtract(x=w145, y=w144) -> (x-y=w143:u16)
            n208 = Subtract "The error"(x=w143, y=w142) -> (x-y=w120:u16)
            n209 = case shown="1, Default" w185 {
              tunnel: ["DIO count 1 (ticks)" "DIO count 2 (ticks)" "DIO count 3 (ticks)"] -> w141
              frame 1, Default {
              }
              frame 2 {
              }
              frame 3 {
              }
            }
            n210 = Number To Boolean Array(number=w120) -> (Boolean array=w121:bool[])
            n211 = Or Array Elements(Boolean array=w121) -> (logical OR=w119:bool)
            n212 = Boolean To (0,1)(Boolean=w119) -> (0, 1=w126:i16)
            n213 = To Unsigned Byte Integer(number=w126) -> (unsigned 8bit integer=w123:u8)
            n214 = feedback #16(u8 0) -> (w124:u8)
            n215 = Add(x=w123, y=w124) -> (x+y=w122:u8)
            "DIO Late Counter" <- w122
            n216 = feedback-in #16(w122) -> ()
            n217 = Subtract(x=w141, y=w120) -> (x-y=w140:u16)
            n218 = Split Number(x=w182) -> (hi(x)=w181:u32, lo(x)=w180:u32)
            n219 = Split Number(x=w171) -> (hi(x)=w176:u32, lo(x)=w175:u32)
            n220 = Boolean To (0,1)(Boolean="+ phase (DIO)") -> (0, 1=w137:i16)
            n221 = Split Number(x=w181) -> (lo(x)=w179:u16)  [unwired: 1 out]
            n222 = Split Number(x=w180) -> (hi(x)=w178:u16, lo(x)=w177:u16)
            n223 = Split Number(x=w176) -> (lo(x)=w174:u16)  [unwired: 1 out]
            n224 = Split Number(x=w175) -> (hi(x)=w173:u16, lo(x)=w172:u16)
            n225 = Split Number(x=w130) -> (hi(x)=w132:u8, lo(x)=w131:u8)
            n226 = Split Number(x=w127) -> (hi(x)=w129:u8, lo(x)=w128:u8)
            n227 = Split Number(x=w179) -> (hi(x)=w169:u8, lo(x)=w168:u8)
            n228 = Split Number(x=w178) -> (hi(x)=w167:u8, lo(x)=w166:u8)
            n229 = Split Number(x=w174) -> (hi(x)=w162:u8, lo(x)=w161:u8)
            n230 = Split Number(x=w177) -> (hi(x)=w165:u8, lo(x)=w164:u8)
            n231 = Split Number(x=w173) -> (hi(x)=w160:u8, lo(x)=w159:u8)
            n232 = Split Number(x=w172) -> (hi(x)=w158:u8, lo(x)=w157:u8)
            n233 = Multiply(x=w137, y="Phase count adjustment (DIO)") -> (x*y=w133:i16)
            n234 = feedback #17(i16 0) -> (w135:i16)
            n235 = Subtract(x=w135, y=w133) -> (x-y=w134:i16)
            "DIO Relative phase" <- w134
            n236 = feedback-in #17(w134) -> ()
            n237 = Add(x=w140, y=w133) -> (x+y=w139:u16)
            n238 = Build Array "BD 1 A Stack"(w132, w131) -> (w154:u8[])
            n239 = Build Array "BD 2 A Stack"(w129, w128) -> (w153:u8[])
            n240 = Build Array "BD 1 nu Stack"(w169, w168, w167, w166, w165, w164) -> (w163:u8[])
            n241 = Build Array "BD 2 nu Stack"(w162, w161, w160, w159, w158, w157) -> (w156:u8[])
            n242 = case shown="2" w170 {
              tunnel: [w225 w228] -> w152
              tunnel: [u8 10 u8 4] -> w155
              tunnel: "Swap F1 and F2" -> [w226 w228]
              frame 2 {
                # "F2"
                n243 = Not(x=w226) -> (.not. x?=w225:bool)
              }
              frame 1, Default {
                # "low chooses F1"
                # "F1"
              }
            }
            n244 = case "If FPGA is controlling (toggling) RF synth" shown="True" w151 {
              tunnel: w163 -> [_ w201]
              tunnel: w156 -> [_ w200]
              tunnel: w155 -> [_ w199]
              tunnel: w154 -> [_ w198]
              tunnel: w153 -> [_ w197]
              frame False {
              }
              frame True {
                # "Write next amp.\n(wait until beginning of next loop iteration to update)"
                n245 = flat-sequence "Update the next F1 and F2 frequency value (the actual frequency won't change until FSK is switched).\nThen load the next amplitude value into buffer, but don't update it until the next cycle." {
                  tunnel: w200 -> [w203]
                  tunnel: w201 -> [w204]
                  tunnel: [w204] -> w196
                  tunnel: [w203] -> w195
                  tunnel: w199 -> [w205]
                  tunnel: w196 -> [w207]
                  tunnel: w195 -> [w206]
                  tunnel: w198 -> [w218]
                  tunnel: w197 -> [w217]
                  frame #0 {
                    # "To possibly send\nthese writes to very\nend of loop (for x and\ny phase adjust)"
                    n246 = call "Wait8"("Count(Ticks)"="Next trap write delay (ticks)") -> ()  [unwired: 1 out]
                  }
                  frame #1 {
                    n247 = for {
                      tunnel: w207 -> [w213] mode=indexing
                      tunnel: w206 -> [w212] mode=indexing
                      tunnel: w205 -> [w210]
                      i -> [w211]
                      # "Write next freq."
                      n248 = To Unsigned Byte Integer(number=w211) -> (unsigned 8bit integer=w208:u8)
                      n249 = Add(x=w210, y=w208) -> (x+y=w209:u8)
                      n250 = call "write to RF synth bd.vi"("Address Byte"=w209, "BD 2 Byte"=w212, "BD 1 Byte"=w213) -> ()
                    }
                  }
                  frame #2 {
                    w214 = TRUE ("Connector1/DIO15")
                    # "send udclk high\n(BD 1 and 2)"
                    n251 = xnode "FPGA I/O Node"("Connector1/DIO30"=w214, "Connector1/DIO29"=w214) -> ()  [unwired: 2 in, 2 out]
                  }
                  frame #3 {
                    w215 = FALSE ("Connector1/DIO15")
                    n252 = xnode "FPGA I/O Node"("Connector1/DIO30"=w215, "Connector1/DIO29"=w215) -> ()  [unwired: 2 in, 2 out]
                  }
                  frame #4 {
                    n253 = for {
                      tunnel: w218 -> [w224] mode=indexing
                      tunnel: w217 -> [w223] mode=indexing
                      tunnel: u8 33 -> [w221]
                      i -> [w222]
                      n254 = To Unsigned Byte Integer(number=w222) -> (unsigned 8bit integer=w219:u8)
                      n255 = Add(x=w221, y=w219) -> (x+y=w220:u8)
                      n256 = call "write to RF synth bd.vi"("Address Byte"=w220, "BD 2 Byte"=w223, "BD 1 Byte"=w224) -> ()
                    }
                  }
                }
              }
            }
          }
        }
      }
    }
  }
  n257 = while "RF box board direct communication loop" {
    tunnel: w2 -> [_]
    stop <- FALSE stop-if-true
    n258 = case "Whether to use direct communication method (only use one method at a time)" shown="True" "Direct RF Box \nCommunication" {
      frame False {
      }
      frame True {
        n259 = case shown="True" "Update Data" {
          frame False {
          }
          frame True {
            n260 = flat-sequence {
              frame #0 {
                n261 = First Call?() -> (First Call?: T/F=w478:bool)
                n262 = case shown="True" w478 {
                  frame False {
                  }
                  frame True {
                    # "If first time data updated, be sure to set WR high\nbefore setting data and address bits."
                    n263 = flat-sequence {
                      frame #0 {
                        n264 = xnode "FPGA I/O Node"("Connector1/DIO15"=TRUE) -> ()  [unwired: 1 in, 1 out]
                      }
                      frame #1 {
                        n265 = call "Wait"("Count(Ticks)"=u8 40 ("DO Delay 3 (Ticks)")) -> ()  [unwired: 1 out]
                      }
                    }
                  }
                }
              }
              frame #1 {
                n266 = Number To Boolean Array(number="Address") -> (Boolean array=w527:bool[])
                n267 = Number To Boolean Array(number="Data BD 1") -> (Boolean array=w528:bool[])
                n268 = Number To Boolean Array(number="Data BD 2") -> (Boolean array=w497:bool[])
                n269 = Index Array(array=w528, index=7) -> (element=w512:bool)
                n270 = Index Array(array=w528, index=6) -> (element=w511:bool)
                n271 = Index Array(array=w528, index=5) -> (element=w510:bool)
                n272 = Index Array(array=w528, index=4) -> (element=w509:bool)
                n273 = Index Array(array=w528, index=3) -> (element=w508:bool)
                n274 = Index Array(array=w528, index=2) -> (element=w507:bool)
                n275 = Index Array(array=w528, index=1) -> (element=w506:bool)
                n276 = Index Array(array=w528, index=0) -> (element=w505:bool)
                n277 = Index Array(array=w527, index=5) -> (element=w504:bool)
                n278 = Index Array(array=w527, index=4) -> (element=w503:bool)
                n279 = Index Array(array=w527, index=3) -> (element=w502:bool)
                n280 = Index Array(array=w527, index=2) -> (element=w501:bool)
                n281 = Index Array(array=w527, index=1) -> (element=w500:bool)
                n282 = Index Array(array=w527, index=0) -> (element=w499:bool)
                n283 = Index Array(array=w497, index=7) -> (element=w488:bool)
                n284 = Index Array(array=w497, index=6) -> (element=w487:bool)
                n285 = Index Array(array=w497, index=5) -> (element=w486:bool)
                n286 = Index Array(array=w497, index=4) -> (element=w485:bool)
                n287 = Index Array(array=w497, index=3) -> (element=w484:bool)
                n288 = Index Array(array=w497, index=2) -> (element=w483:bool)
                n289 = Index Array(array=w497, index=1) -> (element=w482:bool)
                n290 = Index Array(array=w497, index=0) -> (element=w481:bool)
                n291 = xnode "FPGA I/O Node"("Connector1/DIO0"=w512, "Connector1/DIO1"=w511, "Connector1/DIO2"=w510, "Connector1/DIO3"=w509, "Connector1/DIO4"=w508, "Connector1/DIO5"=w507, "Connector1/DIO6"=w506, "Connector1/DIO7"=w505, "Connector1/DIO8"=w504, "Connector1/DIO9"=w503, "Connector1/DIO10"=w502, "Connector1/DIO11"=w501, "Connector1/DIO12"=w500, "Connector1/DIO13"=w499, "Connector1/DIO20"=w488, "Connector1/DIO21"=w487, "Connector1/DIO22"=w486, "Connector1/DIO23"=w485, "Connector1/DIO24"=w484, "Connector1/DIO25"=w483, "Connector1/DIO26"=w482, "Connector1/DIO27"=w481) -> ()  [unwired: 22 in, 22 out]
              }
              frame #2 {
                # "wait and then apply write signal"
                n292 = call "Wait2"("Count(Ticks)"=u8 40 ("DO Delay 1 (Ticks)")) -> ()  [unwired: 1 out]
              }
              frame #3 {
                # "sending bit low writes data to board buffer"
                n293 = xnode "FPGA I/O Node"("Connector1/DIO15"=FALSE) -> ()  [unwired: 1 in, 1 out]
              }
              frame #4 {
                # "wait then return write signal"
                n294 = call "Wait3"("Count(Ticks)"=u8 40 ("DO Delay 2 (Ticks)")) -> ()  [unwired: 1 out]
              }
              frame #5 {
                # "sending bit high makes ready to\nwrite more data"
                n295 = xnode "FPGA I/O Node"("Connector1/DIO15"=TRUE) -> ()  [unwired: 1 in, 1 out]
              }
            }
          }
        }
      }
    }
  }
  n296 = while {
    shift-right: [w536] -> _
    shift-left: FPGAHandShakeState."Wait Ready" ("f") -> [w537]
    stop <- FALSE stop-if-true
    # "Write"
    n297 = case shown="\"ReadWrite\"" w537 {
      tunnel: [w538 FPGAHandShakeState."UnSet Ready" ("f") FPGAHandShakeState."Wait Ready" ("f")] -> w536
      frame "Wait Ready", Default {
        n298 = Select(t=FPGAHandShakeState."ReadWrite" ("Enum"), s="Ready Write", f=FPGAHandShakeState."Wait Ready") -> (s? t:f=w538:T3)
      }
      frame "ReadWrite" {
        n299 = xnode ("Memory Method Node")("Address"="Address 2", "Data"="Data", "Memory In"=refnum<k21> "Trap osc memory") -> ()  [unwired: 1 out]
      }
      frame "UnSet Ready" {
        n300 = local write "Ready Write"(FALSE ("Ready Read")) -> ()
      }
    }
  }
  n301 = To Unsigned Long Integer(number=w2) -> (unsigned 32bit integer=w7:u32)
  n302 = while "APD 1 Counter" {
    tunnel: w2 -> [_]
    stop <- FALSE stop-if-true
    n303 = flat-sequence {
      frame #0 {
        n304 = xnode "FPGA I/O Method Node"("FPGA I/O In"=refnum<k21> "Connector0/DIO0" ("APD 1 DO"), "Timeout"=-1) -> ()  [unwired: 2 out]
      }
      frame #1 {
        n305 = local read "APD1 out state"() -> (w551:bool)
        n306 = case shown="False" w551 {
          frame False {
            n307 = local read "APD 1 Counts 0"() -> (w553:u32)
            n308 = Increment(x=w553) -> (x+1=→"APD 1 Counts 0":u32)
          }
          frame True {
            n309 = local read "APD 1 Counts 1"() -> (w555:u32)
            n310 = Increment(x=w555) -> (x+1=→"APD 1 Counts 1":u32)
          }
        }
      }
    }
  }
  n311 = while "APD 2 Counter" {
    tunnel: w2 -> [_]
    stop <- FALSE stop-if-true
    n312 = flat-sequence {
      frame #0 {
        n313 = xnode "FPGA I/O Method Node"("FPGA I/O In"=refnum<k21> "Connector0/DIO1" ("APD 2 DO"), "Timeout"=-1) -> ()  [unwired: 2 out]
      }
      frame #1 {
        n314 = local read "APD2 out state"() -> (w559:bool)
        n315 = case shown="False" w559 {
          frame False {
            n316 = local read "APD 2 Counts 0"() -> (w561:u32)
            n317 = Increment(x=w561) -> (x+1=→"APD 2 Counts 0":u32)
          }
          frame True {
            n318 = local read "APD 2 Counts 1"() -> (w563:u32)
            n319 = Increment(x=w563) -> (x+1=→"APD 2 Counts 1":u32)
          }
        }
      }
    }
  }
  n320 = while "APD 2 Gating" {
    shift-right: [w567] -> _
    shift-left: w2 -> [w572]
    shift-right: [w566] -> _
    shift-left: w6 -> [w564]
    stop <- FALSE stop-if-true
    n321 = flat-sequence {
      tunnel: w572 -> [w575]
      tunnel: [w576] -> w570
      tunnel: [w575] -> w568
      tunnel: [w574] -> w565
      tunnel: w564 -> [w574]
      tunnel: [w579] -> w571
      tunnel: w570 -> [w579]
      tunnel: [w578] -> w569
      tunnel: w568 -> [w578]
      tunnel: w565 -> [w577]
      tunnel: [w597] -> w567
      tunnel: w571 -> [w608]
      tunnel: w569 -> [w606]
      tunnel: [w601] -> w566
      frame #0 {
        n322 = call "Loop Timer8"("Count(Ticks)"=w575) -> ("Tick Count(Ticks)"=w576:u16)
      }
      frame #1 {
        # "Signal is then sent through \na transistor before APD"
        n323 = xnode "FPGA I/O Node"("Connector0/DIO8"=w577) -> ()  [unwired: 1 in, 1 out]
      }
      frame #2 {
        n324 = local read "APD Gate ON Count"() -> (w590:u16)
        n325 = local read "APD Gate OFF Count"() -> (w589:u16)
        n326 = feedback #18(TRUE) -> (w603:bool)
        n327 = feedback-in #19(w608) -> ()
        n328 = feedback #19(w608) -> (w591:u16)
        n329 = Not(x=w603) -> (.not. x?=w600:bool)
        n330 = feedback-in #18(w600) -> ()
        n331 = Subtract(x=w608, y=w591) -> (x-y=w607:u16)
        n332 = Select(t=w590, s=w600, f=w589) -> (s? t:f=w605:u16)
        n333 = Subtract(x=w607, y=w606) -> (x-y=w582:u16)
        n334 = Subtract(x=w605, y=w582) -> (x-y=w596:u16)
        n335 = Number To Boolean Array(number=w582) -> (Boolean array=w581:bool[])
        n336 = Or Array Elements(Boolean array=w581) -> (logical OR=w580:bool)
        n337 = Boolean To (0,1)(Boolean="+ phase (APD 2 Gate)") -> (0, 1=w594:i16)
        n338 = Multiply(x=w594, y="Phase count adjustment (APD 2 Gate)") -> (x*y=w592:i16)
        n339 = Boolean To (0,1)(Boolean=w580) -> (0, 1=w587:i16)
        n340 = Add(x=w596, y=w592) -> (x+y=w597:u16)
        n341 = To Unsigned Byte Integer(number=w587) -> (unsigned 8bit integer=w584:u8)
        n342 = feedback #20(i16 0) -> (w599:i16)
        n343 = Subtract(x=w599, y=w592) -> (x-y=w598:i16)
        "APD 2 Gate Relative Phase" <- w598
        n344 = feedback-in #20(w598) -> ()
        n345 = feedback #21(u8 0) -> (w585:u8)
        n346 = Add(x=w584, y=w585) -> (x+y=w583:u8)
        "APD 2 Gate Late Counter" <- w583
        n347 = feedback-in #21(w583) -> ()
        n348 = local read "APD Gate Operating Mode"() -> (w588:u8)
        n349 = case shown="2" w588 {
          tunnel: [TRUE FALSE w614] -> w601
          tunnel: w603 -> [_ _ w612]
          frame 0, Default {
          }
          frame 1 {
          }
          frame 2 {
            n350 = local read "Invert APD Gate"() -> (w611:bool)
            n351 = Not(x=w612) -> (.not. x?=w613:bool)
            n352 = Select(t=w613, s=w611, f=w612) -> (s? t:f=w614:bool)
          }
        }
      }
    }
  }
  n353 = while "532 nm green fluorescent laser interlacing (DO to IA 532 nm AOM ME amp)." {
    shift-right: [w618] -> _
    shift-left: w2 -> [w623]
    shift-right: [w617] -> _
    shift-left: w3 -> [w615]
    stop <- FALSE stop-if-true
    n354 = flat-sequence {
      tunnel: w623 -> [w626]
      tunnel: [w627] -> w621
      tunnel: [w626] -> w619
      tunnel: [w625] -> w616
      tunnel: w615 -> [w625]
      tunnel: [w630] -> w622
      tunnel: w621 -> [w630]
      tunnel: [w629] -> w620
      tunnel: w619 -> [w629]
      tunnel: w616 -> [w628]
      tunnel: [w639] -> w618
      tunnel: w622 -> [w659]
      tunnel: w620 -> [w656]
      tunnel: [w648] -> w617
      frame #0 {
        n355 = call "Loop Timer4"("Count(Ticks)"=w626) -> ("Tick Count(Ticks)"=w627:u16)
      }
      frame #1 {
        # "Then to PRL 440 amp"
        n356 = xnode "FPGA I/O Node"("Connector1/DIO39"=w628) -> ()  [unwired: 1 in, 1 out]
      }
      frame #2 {
        n357 = feedback-in #22(w659) -> ()
        n358 = feedback #22(w659) -> (w658:u16)
        n359 = Subtract(x=w659, y=w658) -> (x-y=w657:u16)
        n360 = Subtract(x=w657, y=w656) -> (x-y=w632:u16)
        n361 = Number To Boolean Array(number=w632) -> (Boolean array=w633:bool[])
        n362 = Or Array Elements(Boolean array=w633) -> (logical OR=w631:bool)
        n363 = Boolean To (0,1)(Boolean="+ phase (GI)") -> (0, 1=w644:i16)
        n364 = Multiply(x=w644, y="Phase count adjustment (GI)") -> (x*y=w641:i16)
        n365 = Boolean To (0,1)(Boolean=w631) -> (0, 1=w638:i16)
        n366 = To Unsigned Byte Integer(number=w638) -> (unsigned 8bit integer=w635:u8)
        n367 = feedback #23(i16 0) -> (w642:i16)
        n368 = feedback #24(u8 0) -> (w636:u8)
        n369 = Add(x=w635, y=w636) -> (x+y=w634:u8)
        "GI Late Counter" <- w634
        n370 = feedback-in #24(w634) -> ()
        n371 = Subtract(x=w642, y=w641) -> (x-y=w640:i16)
        "GI Relative phase" <- w640
        n372 = feedback-in #23(w640) -> ()
        n373 = feedback #25(TRUE) -> (w651:bool)
        n374 = case shown="2" "Operating Mode" {
          tunnel: [TRUE FALSE w665] -> w648
          tunnel: w651 -> [_ _ w662]
          frame 0, Default {
          }
          frame 1 {
          }
          frame 2 {
            n375 = Not(x=w662) -> (.not. x?=w664:bool)
            n376 = Select(t=w664, s="Invert GI", f=w662) -> (s? t:f=w665:bool)
          }
        }
        n377 = Not(x=w651) -> (.not. x?=w647:bool)
        n378 = Select(t="Green interlace ON count", s=w647, f="Green interlace OFF count") -> (s? t:f=w653:u16)
        n379 = Subtract(x=w653, y=w632) -> (x-y=w645:u16)
        n380 = Add(x=w645, y=w641) -> (x+y=w639:u16)
        n381 = feedback-in #25(w647) -> ()
      }
    }
  }
  n382 = while "Green and red fluorescent laser interlacing (Current AO to IA 532 nm AOM ME amp)." {
    shift-right: [w674] -> _
    shift-left: w2 -> [w677]
    shift-right: [w671] -> _
    shift-left: w4 -> [w669]
    shift-right: [w668] -> _
    shift-left: w4 -> [w667]
    stop <- FALSE stop-if-true
    n383 = flat-sequence {
      tunnel: w677 -> [w681]
      tunnel: [w682] -> w676
      tunnel: [w681] -> w675
      tunnel: [w680] -> w670
      tunnel: w669 -> [w680]
      tunnel: w667 -> [w679]
      tunnel: [w679] -> w666
      tunnel: [w686] -> w673
      tunnel: w676 -> [w686]
      tunnel: [w685] -> w672
      tunnel: w675 -> [w685]
      tunnel: w670 -> [w684]
      tunnel: w666 -> [w683]
      tunnel: [w707] -> w674
      tunnel: [w723] -> w671
      tunnel: w673 -> [w734]
      tunnel: w672 -> [w731]
      tunnel: [w691] -> w668
      frame #0 {
        n384 = call "Loop Timer10"("Count(Ticks)"=w681) -> ("Tick Count(Ticks)"=w682:u16)
      }
      frame #1 {
        n385 = xnode "FPGA I/O Node"("Chassis2/Mod4/AO0"=w684, "Chassis2/Mod4/AO1"=w683) -> ()  [unwired: 2 in, 2 out]
      }
      frame #2 {
        # "Design note:\n\nThese two laser controls are in the same loop\nbecause the expansion current AI cannot separately\ntime the outputs fast enough for us.  Apparently\nit is because of communication time between the\nexpansion card and the fpga.\n\nSo the two analog control signals have the same timing\nand profile, but independent amplitudes to independently\ncontrol the intensity and feedback for each laser."
        n386 = feedback #26(TRUE) -> (w687:bool)
        n387 = Not(x=w687) -> (.not. x?=w688:bool)
        n388 = feedback-in #26(w688) -> ()
        n389 = Subtract(x="Green interlace OFF count 2", y="Green int current ON count adj") -> (x-y=w716:u16)
        n390 = feedback-in #27(w734) -> ()
        n391 = feedback #27(w734) -> (w733:u16)
        n392 = Add(x="Green int current ON count adj", y="Green interlace ON count 2") -> (x+y=w717:u16)
        n393 = Subtract(x=w734, y=w733) -> (x-y=w732:u16)
        n394 = Select(t=w717, s=w688, f=w716) -> (s? t:f=w728:u16)
        n395 = Subtract(x=w732, y=w731) -> (x-y=w700:u16)
        n396 = case shown="2" "RI Operating Mode 2" {
          tunnel: [TRUE FALSE w740] -> w689
          tunnel: w687 -> [_ _ w737]
          frame 0, Default {
          }
          frame 1 {
          }
          frame 2 {
            n397 = Not(x=w737) -> (.not. x?=w739:bool)
            n398 = Select(t=w739, s="Invert RI 2", f=w737) -> (s? t:f=w740:bool)
          }
        }
        n399 = Subtract(x=w728, y=w700) -> (x-y=w711:u16)
        n400 = case shown="0, Default" "Operating Mode 2" {
          tunnel: [TRUE FALSE w774] -> w692
          tunnel: w687 -> [_ _ w771]
          frame 0, Default {
          }
          frame 1 {
          }
          frame 2 {
            n401 = Not(x=w771) -> (.not. x?=w773:bool)
            n402 = Select(t=w773, s="Invert GI 2", f=w771) -> (s? t:f=w774:bool)
          }
        }
        n403 = Number To Boolean Array(number=w700) -> (Boolean array=w701:bool[])
        n404 = Boolean To (0,1)(Boolean="+ phase (GI) 2") -> (0, 1=w713:i16)
        n405 = Or Array Elements(Boolean array=w701) -> (logical OR=w699:bool)
        n406 = Boolean To (0,1)(Boolean=w699) -> (0, 1=w706:i16)
        n407 = Multiply(x=w713, y="Phase count adjustment (GI) 2") -> (x*y=w709:i16)
        n408 = To Unsigned Byte Integer(number=w706) -> (unsigned 8bit integer=w702:u8)
        n409 = Add(x=w711, y=w709) -> (x+y=w707:u16)
        n410 = feedback #28(u8 0) -> (w704:u8)
        n411 = Add(x=w702, y=w704) -> (x+y=w703:u8)
        "GI Late Counter 2" <- w703
        n412 = feedback-in #28(w703) -> ()
        n413 = feedback #29(i16 0) -> (w710:i16)
        n414 = Subtract(x=w710, y=w709) -> (x-y=w708:i16)
        "GI Relative phase 2" <- w708
        n415 = feedback-in #29(w708) -> ()
        n416 = And(x=w692, y="Green FB On/Off") -> (x .and. y?=w718:bool)
        n417 = And(x=w689, y="Red FB On/Off") -> (x .and. y?=w698:bool)
        n418 = case shown="True" w718 {
          tunnel: "Current Out" -> [w755 _]
          tunnel: [w755 w764] -> w722
          frame False {
          }
          frame True {
            n419 = local read "Green FB Sum"() -> (w760:i16)
            n420 = Bundle("P3"="P3", "I3"="I3", "D3"="D3") -> (w756:cluster{"P3":i16, "I3":i16, "D3":i16})  [unwired: 1 in]
            n421 = call "Slower PID.vi"("process variable"=w760, "reset?"="Green FB Reset", "setpoint"="Green FB Setpoint", "PID gains (x 2^8)"=w756, "output range"=cluster{"output high":i16, "output low":i16} {"output high"=32767, "output low"=-32768} ("Green FB output range")) -> ("output"=w767:i16)  [unwired: 10 out]
            n422 = To Long Integer(number=w767) -> (32bit integer=w761:i32)
            n423 = Add(x=w761, y=32768) -> (x+y=w763:i32)
            n424 = To Unsigned Word Integer(number=w763) -> (unsigned 16bit integer=w764:u16)
          }
        }
        n425 = case shown="True" w698 {
          tunnel: "RI Current Out" -> [w741 _]
          tunnel: [w741 w750] -> w694
          frame False {
          }
          frame True {
            n426 = local read "Red FB Intensity"() -> (w746:i16)
            n427 = Bundle("P4"="P4", "I4"="I4", "D4"="D4") -> (w742:cluster{"P4":i16, "I4":i16, "D4":i16})  [unwired: 1 in]
            n428 = call "Slower PID.vi"("process variable"=w746, "reset?"="Red FB Reset", "setpoint"="Red FB Setpoint", "PID gains (x 2^8)"=w742, "output range"=cluster{"output high":i16, "output low":i16} {"output high"=32767, "output low"=-32768} ("Green FB output range")) -> ("output"=w753:i16)  [unwired: 10 out]
            n429 = To Long Integer(number=w753) -> (32bit integer=w747:i32)
            n430 = Add(x=w747, y=32768) -> (x+y=w749:i32)
            n431 = To Unsigned Word Integer(number=w749) -> (unsigned 16bit integer=w750:u16)
          }
        }
        n432 = Boolean To (0,1)(Boolean=w692) -> (0, 1=w724:i16)
        n433 = Boolean To (0,1)(Boolean=w689) -> (0, 1=w693:i16)
        n434 = To Unsigned Word Integer(number=w724) -> (unsigned 16bit integer=w721:u16)
        n435 = To Unsigned Word Integer(number=w693) -> (unsigned 16bit integer=w695:u16)
        n436 = Multiply(x=w721, y=w722) -> (x*y=w723:u16)
        n437 = Multiply(x=w695, y=w694) -> (x*y=w691:u16)
      }
    }
  }
  n438 = while "MCL stage control" {
    shift-right: [w787] -> _
    shift-left: w2 -> [w790]
    shift-right: [w780] -> _
    shift-left: w11 -> [w777]
    shift-right: [w779] -> _
    shift-left: w10 -> [w775]
    stop <- FALSE stop-if-true
    n439 = flat-sequence {
      tunnel: w790 -> [w794]
      tunnel: [w795] -> w786
      tunnel: [w794] -> w784
      tunnel: [w793] -> w778
      tunnel: w777 -> [w793]
      tunnel: [w792] -> w776
      tunnel: w775 -> [w792]
      tunnel: w786 -> [w799]
      tunnel: [w799] -> w785
      tunnel: w784 -> [w798]
      tunnel: [w798] -> w783
      tunnel: w778 -> [w797]
      tunnel: w776 -> [w796]
      tunnel: w785 -> [w807]
      tunnel: w783 -> [w806]
      tunnel: [w807] -> w789
      tunnel: [w806] -> w788
      tunnel: [w805] -> w782
      tunnel: [w804] -> w781
      tunnel: [w879] -> w787
      tunnel: w789 -> [w886]
      tunnel: w788 -> [w883]
      tunnel: w782 -> [w881]
      tunnel: w781 -> [w880]
      tunnel: [w881] -> w780
      tunnel: [w880] -> w779
      frame #0 {
        n440 = call "Loop Timer5"("Count(Ticks)"=w794) -> ("Tick Count(Ticks)"=w795:u32)
      }
      frame #1 {
        n441 = xnode "FPGA I/O Node"("Connector0/AO1"=w797, "Connector0/AO2"=w796) -> ()  [unwired: 2 in, 2 out]
      }
      frame #2 {
        n442 = local read "Scanning MCL"() -> (w819:bool)
        n443 = Or(x=w819, y="Start scan (MCL)") -> (x .or. y?=w814:bool)
        n444 = Not(x="Abort scan (MCL)") -> (.not. x?=w812:bool)
        n445 = And(x=w812, y=w814) -> (x .and. y?=w811:bool)
        n446 = case "Raster scan" shown="True" w811 {
          tunnel: [w820 w863] -> w816
          tunnel: "Start scan (MCL)" -> [_ w848]
          tunnel: [w820 w824] -> w800
          frame False {
            w820 = i16 0
            n447 = local write "Scanning MCL"(FALSE ("scanning")) -> ()
          }
          frame True {
            w834 = i16 0
            w833 = u64 0
            # "scan incr."
            # "freq. incr. mult."
            # "count steps"
            # "count number of cycles"
            n448 = feedback #30(w833) -> (w860:u64)
            n449 = Select(t=w833, s=w848, f=w860) -> (s? t:f=w862:u64)
            n450 = Increment(x=w862) -> (x+1=w859:u64)
            n451 = Greater?(x="Cycles per step (MCL)", y=w859) -> (0:w843:bool)
            n452 = Select(t=w859, s=w843, f=w833) -> (s? t:f=w858:u64)
            n453 = feedback-in #30(w858) -> ()
            n454 = feedback #31(w833) -> (w857:u64)
            n455 = Select(t=w833, s=w848, f=w857) -> (s? t:f=w852:u64)
            n456 = Increment(x=w852) -> (x+1=w856:u64)
            n457 = Add(x="Scan steps (MCL)", y="Scan steps (MCL)") -> (x+y=w855:u64)
            n458 = Select(t=w852, s=w843, f=w856) -> (s? t:f=w838:u64)
            n459 = Greater?(x=w855, y=w838) -> (0:w837:bool)
            n460 = Select(t=w838, s=w837, f=w833) -> (s? t:f=w853:u64)
            n461 = feedback-in #31(w853) -> ()
            n462 = Equal?(x="Scan steps (MCL)", y=w838) -> (x = y?=w842:bool)
            n463 = Greater?(x="Scan steps (MCL)", y=w852) -> (0:w851:bool)
            n464 = feedback #32(w834) -> (w854:i16)
            n465 = Select(t=w834, s=w848, f=w854) -> (s? t:f=w840:i16)
            n466 = Increment(x=w840) -> (x+1=w850:i16)
            n467 = Decrement(x=w840) -> (x-1=w849:i16)
            n468 = Select(t=w850, s=w851, f=w849) -> (s? t:f=w841:i16)
            n469 = Select(t=w840, s=w842, f=w841) -> (s? t:f=w839:i16)
            n470 = Select(t=w840, s=w843, f=w839) -> (s? t:f=w835:i16)
            n471 = Select(t=w835, s=w837, f=w834) -> (s? t:f=w836:i16)
            n472 = feedback-in #32(w836) -> ()
            n473 = feedback #33(w833) -> (w847:u64)
            n474 = Select(t=w833, s=w848, f=w847) -> (s? t:f=w822:u64)
            n475 = Increment(x=w822) -> (x+1=w844:u64)
            n476 = Select(t=w822, s=w837, f=w844) -> (s? t:f=w823:u64)
            n477 = Greater?(x="Number of scans (MCL)", y=w823) -> (0:w830:bool)
            n478 = Multiply(x="Scan freq.  increment (MCL)", y=w840) -> (x*y=w863:i16)
            n479 = Select(t=TRUE, s="Cont. Scan (MCL)", f=w830) -> (s? t:f=w829:bool)
            "Scanning MCL" <- w829
            n480 = Select(t=w823, s=w829, f=w833) -> (s? t:f=w845:u64)
            n481 = feedback-in #33(w845) -> ()
            n482 = Increment(x=w823) -> (x+1=→"Scan I (MCL)":u64)
            n483 = To Word Integer(number=w822) -> (16bit integer=w825:i16)
            n484 = Multiply(x=w825, y="Scan freq.  increment (MCL)") -> (x*y=w824:i16)
          }
        }
        n485 = Select(t=w800, s="1D or 2D Scan?", f=i16 0) -> (s? t:f=w801:i16)
        n486 = Select(t=w801, s="MCL Scan Axis", f=w816) -> (s? t:f=w815:i16)
        n487 = Select(t=w816, s="MCL Scan Axis", f=w801) -> (s? t:f=w817:i16)
        n488 = Add(x=w815, y="AO2") -> (x+y=w804:i16)
        n489 = Add(x="AO1", y=w817) -> (x+y=w805:i16)
      }
      frame #3 {
        n490 = feedback-in #34(w886) -> ()
        n491 = feedback #34(w886) -> (w885:u32)
        n492 = Boolean To (0,1)(Boolean="+ phase (MCL)") -> (0, 1=w877:i16)
        n493 = Subtract(x=w886, y=w885) -> (x-y=w884:u32)
        n494 = Multiply(x=w877, y="Phase count adjustment (MCL)") -> (x*y=w873:i16)
        n495 = Subtract(x=w884, y=w883) -> (x-y=w865:u32)
        n496 = Subtract(x="MCL count", y=w865) -> (x-y=w875:u32)
        n497 = feedback #35(i16 0) -> (w874:i16)
        n498 = Subtract(x=w874, y=w873) -> (x-y=w872:i16)
        "MCL Relative Phase" <- w872
        n499 = feedback-in #35(w872) -> ()
        n500 = Number To Boolean Array(number=w865) -> (Boolean array=w866:bool[])
        n501 = Or Array Elements(Boolean array=w866) -> (logical OR=w864:bool)
        n502 = Boolean To (0,1)(Boolean=w864) -> (0, 1=w871:i16)
        n503 = Add(x=w875, y=w873) -> (x+y=w879:u32)
        n504 = To Unsigned Byte Integer(number=w871) -> (unsigned 8bit integer=w868:u8)
        n505 = feedback #36(u8 0) -> (w869:u8)
        n506 = Add(x=w868, y=w869) -> (x+y=w867:u8)
        "MCL Late Counter" <- w867
        n507 = feedback-in #36(w867) -> ()
      }
    }
  }
  n508 = while "Excitation laser intensity feedback measurement (all lasers)" {
    shift-right: [w888] -> _
    shift-left: w2 -> [w893]
    stop <- FALSE stop-if-true
    n509 = flat-sequence {
      tunnel: w893 -> [w895]
      tunnel: [w896] -> w891
      tunnel: [w895] -> w889
      tunnel: [w902] -> w892
      tunnel: w891 -> [w902]
      tunnel: [w901] -> w890
      tunnel: w889 -> [w901]
      tunnel: [w914] -> w888
      tunnel: w892 -> [w925]
      tunnel: w890 -> [w922]
      frame #0 {
        n510 = call "Loop Timer9"("Count(Ticks)"=w895) -> ("Tick Count(Ticks)"=w896:u16)
      }
      frame #1 {
        # "Design note:\n\nAll lasers need to be measured at the same \ntime because the AI expansion module\ncannot independently time the measurements\nwithin our requirements: their is dead time.\n\nThis probably wouldn't be an issue with the built\nin AI on the fpga board itself."
        n511 = xnode "FPGA I/O Node"("Connector1/DIO35"=TRUE) -> ("Chassis2/Mod1/AI2"=→"Blue Intensity":i16, "Chassis2/Mod1/AI1"=→"Red FB Intensity":i16, "Chassis2/Mod1/AI0"=→"Green FB Sum":i16)  [unwired: 4 in, 4 out]
      }
      frame #2 {
        n512 = feedback-in #37(w925) -> ()
        n513 = feedback #37(w925) -> (w924:u16)
        n514 = Subtract(x=w925, y=w924) -> (x-y=w923:u16)
        n515 = xnode "FPGA I/O Node"("Connector1/DIO35"=FALSE) -> ()  [unwired: 1 in, 1 out]
        n516 = Subtract(x=w923, y=w922) -> (x-y=w904:u16)
        n517 = Subtract(x="Green FB Count", y=w904) -> (x-y=w918:u16)
        n518 = Number To Boolean Array(number=w904) -> (Boolean array=w905:bool[])
        n519 = Or Array Elements(Boolean array=w905) -> (logical OR=w903:bool)
        n520 = Boolean To (0,1)(Boolean="+ phase (Green FB)") -> (0, 1=w916:i16)
        n521 = Boolean To (0,1)(Boolean=w903) -> (0, 1=w910:i16)
        n522 = Multiply(x=w916, y="Phase count adjustment (Green FB)") -> (x*y=w911:i16)
        n523 = Add(x=w918, y=w911) -> (x+y=w914:u16)
        n524 = To Unsigned Byte Integer(number=w910) -> (unsigned 8bit integer=w907:u8)
        n525 = feedback #38(i16 0) -> (w913:i16)
        n526 = Subtract(x=w913, y=w911) -> (x-y=w912:i16)
        "Green FB Relative Phase" <- w912
        n527 = feedback-in #38(w912) -> ()
        n528 = feedback #39(u8 0) -> (w908:u8)
        n529 = Add(x=w907, y=w908) -> (x+y=w906:u8)
        "Green Late Counter" <- w906
        n530 = feedback-in #39(w906) -> ()
      }
    }
  }
  n531 = while "APD 1 Gating" {
    shift-right: [w929] -> _
    shift-left: w2 -> [w934]
    shift-right: [w928] -> _
    shift-left: w6 -> [w926]
    stop <- FALSE stop-if-true
    n532 = flat-sequence {
      tunnel: w934 -> [w937]
      tunnel: [w938] -> w932
      tunnel: [w937] -> w930
      tunnel: [w936] -> w927
      tunnel: w926 -> [w936]
      tunnel: [w941] -> w933
      tunnel: w932 -> [w941]
      tunnel: [w940] -> w931
      tunnel: w930 -> [w940]
      tunnel: w927 -> [w939]
      tunnel: [w955] -> w929
      tunnel: w933 -> [w970]
      tunnel: w931 -> [w967]
      tunnel: [w959] -> w928
      frame #0 {
        n533 = call "Loop Timer7"("Count(Ticks)"=w937) -> ("Tick Count(Ticks)"=w938:u16)
      }
      frame #1 {
        # "Signal is then sent through \na transistor before APD"
        n534 = xnode "FPGA I/O Node"("Connector0/DIO4"=w939) -> ()  [unwired: 1 in, 1 out]
      }
      frame #2 {
        n535 = feedback #40(TRUE) -> (w962:bool)
        n536 = feedback-in #41(w970) -> ()
        n537 = feedback #41(w970) -> (w969:u16)
        n538 = Not(x=w962) -> (.not. x?=w958:bool)
        n539 = feedback-in #40(w958) -> ()
        n540 = Subtract(x=w970, y=w969) -> (x-y=w968:u16)
        n541 = Select(t="APD Gate ON Count", s=w958, f="APD Gate OFF Count") -> (s? t:f=w964:u16)
        n542 = Subtract(x=w968, y=w967) -> (x-y=w943:u16)
        n543 = Subtract(x=w964, y=w943) -> (x-y=w954:u16)
        n544 = Number To Boolean Array(number=w943) -> (Boolean array=w944:bool[])
        n545 = Or Array Elements(Boolean array=w944) -> (logical OR=w942:bool)
        n546 = Boolean To (0,1)(Boolean="+ phase (APD 1 Gate)") -> (0, 1=w952:i16)
        n547 = Boolean To (0,1)(Boolean=w942) -> (0, 1=w949:i16)
        n548 = Multiply(x=w952, y="Phase count adjustment (APD 1 Gate)") -> (x*y=w950:i16)
        n549 = To Unsigned Byte Integer(number=w949) -> (unsigned 8bit integer=w946:u8)
        n550 = Add(x=w954, y=w950) -> (x+y=w955:u16)
        n551 = feedback #42(i16 0) -> (w957:i16)
        n552 = Subtract(x=w957, y=w950) -> (x-y=w956:i16)
        "APD 1 Gate Relative Phase" <- w956
        n553 = feedback-in #42(w956) -> ()
        n554 = feedback #43(u8 0) -> (w947:u8)
        n555 = Add(x=w946, y=w947) -> (x+y=w945:u8)
        "APD 1 Gate Late Counter" <- w945
        n556 = feedback-in #43(w945) -> ()
        n557 = case shown="2" "APD Gate Operating Mode" {
          tunnel: [TRUE FALSE w976] -> w959
          tunnel: w962 -> [_ _ w973]
          frame 0, Default {
          }
          frame 1 {
          }
          frame 2 {
            n558 = Not(x=w973) -> (.not. x?=w975:bool)
            n559 = Select(t=w975, s="Invert APD Gate", f=w973) -> (s? t:f=w976:bool)
          }
        }
      }
    }
  }
  n560 = while "Control APD data integration - stream to host" {
    shift-right: [w980] -> _
    shift-left: w7 -> [w985]
    stop <- FALSE stop-if-true
    n561 = flat-sequence {
      tunnel: w985 -> [w987]
      tunnel: [w988] -> w983
      tunnel: [w987] -> w981
      tunnel: [w998] -> w984
      tunnel: w983 -> [w998]
      tunnel: [w997] -> w982
      tunnel: w981 -> [w997]
      tunnel: [w996] -> w979
      tunnel: [w995] -> w978
      tunnel: [w989] -> w977
      tunnel: [w1040] -> w980
      tunnel: w984 -> [w1050]
      tunnel: w982 -> [w1047]
      tunnel: w979 -> [w1033]
      tunnel: w978 -> [w1032]
      tunnel: w977 -> [w1020]
      frame #0 {
        n562 = call "Loop Timer6"("Count(Ticks)"=w987) -> ("Tick Count(Ticks)"=w988:u32)
      }
      frame #1 {
        n563 = flat-sequence {
          tunnel: [w1000] -> w994
          tunnel: w994 -> [w1003]
          tunnel: [w1007] -> w993
          tunnel: [w1006] -> w992
          tunnel: [w1003] -> w991
          tunnel: [w1002] -> w990
          tunnel: [w1014] -> w995
          tunnel: [w1015] -> w996
          tunnel: w993 -> [w1015]
          tunnel: w992 -> [w1014]
          tunnel: w991 -> [w1013]
          tunnel: w990 -> [w1012]
          tunnel: [w1012] -> w989
          frame #0 {
            # "use separate variable so each APD won't\nhave to wait to read"
            n564 = feedback #44(FALSE) -> (w999:bool)
            "APD1 out state" <- w999
            "APD2 out state" <- w999
            "APD3 out state" <- w999
            n565 = Not(x=w999) -> (.not. x?=w1000:bool)
            n566 = feedback-in #44(w1000) -> ()
          }
          frame #1 {
            n567 = local read "APD 3 Counts 1"() -> (w1005:u32)
            n568 = local read "APD 3 Counts 0"() -> (w1004:u32)
            n569 = local read "APD 1 Counts 1"() -> (w1011:u32)
            n570 = local read "APD 1 Counts 0"() -> (w1010:u32)
            n571 = local read "APD 2 Counts 1"() -> (w1009:u32)
            n572 = local read "APD 2 Counts 0"() -> (w1008:u32)
            n573 = Select(t=w1005, s=w1003, f=w1004) -> (s? t:f=w1002:u32)
            n574 = Select(t=w1011, s=w1003, f=w1010) -> (s? t:f=w1007:u32)
            n575 = Select(t=w1009, s=w1003, f=w1008) -> (s? t:f=w1006:u32)
          }
          frame #2 {
            n576 = case shown="False" w1013 {
              frame False {
                w1016 = u32 0 ("APD 1 Counts 0")
                n577 = local write "APD 1 Counts 0"(w1016) -> ()
                n578 = local write "APD 2 Counts 0"(w1016) -> ()
                n579 = local write "APD 3 Counts 0"(w1016) -> ()
              }
              frame True {
                w1017 = u32 0 ("APD 1 Counts 1")
                n580 = local write "APD 1 Counts 1"(w1017) -> ()
                n581 = local write "APD 2 Counts 1"(w1017) -> ()
                n582 = local write "APD 3 Counts 1"(w1017) -> ()
              }
            }
          }
        }
      }
      frame #2 {
        n583 = feedback-in #45(w1050) -> ()
        n584 = feedback #45(w1050) -> (w1049:u32)
        n585 = Subtract(x=w1050, y=w1049) -> (x-y=w1048:u32)
        n586 = Subtract(x=w1048, y=w1047) -> (x-y=w1025:u32)
        n587 = case shown="True" "APD to FIFO" {
          tunnel: w1033 -> [_ w1055]
          tunnel: w1032 -> [_ w1053]
          tunnel: w1020 -> [_ w1051]
          frame False {
          }
          frame True {
            n588 = flat-sequence {
              tunnel: 0 ("Timeout") -> [w1057]
              tunnel: w1055 -> [w1058]
              tunnel: [w1057] -> w1054
              tunnel: w1054 -> [w1059]
              tunnel: w1053 -> [w1060]
              tunnel: [w1059] -> w1052
              tunnel: w1052 -> [w1062]
              tunnel: w1051 -> [w1061]
              frame #0 {
                n589 = xnode ("FIFO Write")("Element"=w1058, "Timeout"=w1057) -> ()  [unwired: 1 in, 2 out]
              }
              frame #1 {
                n590 = xnode ("FIFO Write")("Element"=w1060, "Timeout"=w1059) -> ()  [unwired: 1 in, 2 out]
              }
              frame #2 {
                n591 = xnode ("FIFO Write")("Element"=w1061, "Timeout"=w1062) -> ()  [unwired: 1 in, 2 out]
              }
            }
          }
        }
        n592 = Subtract(x="APD Acq Rate Count", y=w1025) -> (x-y=w1041:u32)
        n593 = Number To Boolean Array(number=w1025) -> (Boolean array=w1026:bool[])
        n594 = Or Array Elements(Boolean array=w1026) -> (logical OR=w1024:bool)
        n595 = Boolean To (0,1)(Boolean=w1024) -> (0, 1=w1031:i16)
        n596 = To Unsigned Byte Integer(number=w1031) -> (unsigned 8bit integer=w1028:u8)
        n597 = feedback #46(u8 0) -> (w1029:u8)
        n598 = Add(x=w1028, y=w1029) -> (x+y=w1027:u8)
        "APD Acq Late Counter" <- w1027
        n599 = feedback-in #46(w1027) -> ()
        n600 = Boolean To (0,1)(Boolean="+ phase (APD Acq)") -> (0, 1=w1037:i16)
        n601 = Multiply(x=w1037, y="Phase Count Adjustment (APD Acq)") -> (x*y=w1034:i16)
        n602 = Add(x=w1041, y=w1034) -> (x+y=w1040:u32)
        n603 = feedback #47(i16 0) -> (w1039:i16)
        n604 = Subtract(x=w1039, y=w1034) -> (x-y=w1036:i16)
        "APD Acq Relative Phase" <- w1036
        n605 = feedback-in #47(w1036) -> ()
        n606 = To Word Integer(number=w1033) -> (16bit integer=w1042:i16)
        n607 = To Word Integer(number=w1020) -> (16bit integer=w1021:i16)
        n608 = To Word Integer(number=w1032) -> (16bit integer=w1043:i16)
        n609 = Multiply(x="APD AO scale factor", y=w1043) -> (x*y=w1022:i16)
        n610 = Multiply(x="APD AO scale factor", y=w1021) -> (x*y=w1018:i16)
        n611 = Multiply(x="APD AO scale factor", y=w1042) -> (x*y=w1023:i16)
        n612 = xnode "FPGA I/O Node"("Connector0/AO5"=w1023, "Connector0/AO7"=w1022, "Connector0/AO6"=w1018) -> ()  [unwired: 3 in, 3 out]
      }
    }
  }
  n613 = while "DAQ AI set 1" {
    shift-right: [w1063] -> _
    shift-left: w2 -> [w1068]
    stop <- FALSE stop-if-true
    n614 = flat-sequence {
      tunnel: w1068 -> [w1078]
      tunnel: [w1079] -> w1066
      tunnel: [w1078] -> w1065
      tunnel: [w1089] -> w1076
      tunnel: [w1088] -> w1075
      tunnel: [w1087] -> w1074
      tunnel: [w1086] -> w1073
      tunnel: [w1085] -> w1072
      tunnel: [w1084] -> w1071
      tunnel: [w1083] -> w1070
      tunnel: [w1082] -> w1069
      tunnel: [w1081] -> w1067
      tunnel: w1066 -> [w1081]
      tunnel: w1065 -> [w1080]
      tunnel: [w1080] -> w1064
      tunnel: [w1118] -> w1063
      tunnel: w1076 -> [w1145]
      tunnel: w1075 -> [w1110]
      tunnel: w1074 -> [w1111]
      tunnel: w1073 -> [w1144]
      tunnel: w1072 -> [w1134]
      tunnel: w1071 -> [w1133]
      tunnel: w1070 -> [w1132]
      tunnel: w1069 -> [w1131]
      tunnel: w1067 -> [w1128]
      tunnel: w1064 -> [w1125]
      frame #0 {
        n615 = call "Loop Timer3"("Count(Ticks)"=w1078) -> ("Tick Count(Ticks)"=w1079:u16)
      }
      frame #1 {
        n616 = xnode "FPGA I/O Node"("Connector1/DIO31"=TRUE ("Connector1/DIO33")) -> ("Connector0/AI0"=w1089:i16, "Connector0/AI1"=w1088:i16, "Connector0/AI2"=w1087:i16, "Connector0/AI3"=w1086:i16, "Connector0/AI4"=w1085:i16, "Connector0/AI5"=w1084:i16, "Connector0/AI6"=w1083:i16, "Connector0/AI7"=w1082:i16)  [unwired: 9 in, 9 out]
      }
      frame #2 {
        w1114 = FALSE ("AI to FIFO")
        # "Adjust phase after data acquired if button pressed"
        n617 = feedback #48(i16 1) -> (w1137:i16)
        n618 = Increment(x=w1137) -> (x+1=w1143:i16)
        n619 = Scale By Power Of 2(n="AI1 X Scale", x=w1110) -> (x*2^n=w1108:i16)
        n620 = Greater?(x=w1143, y="N of AI1 Int Acq Sets") -> (0:w1140:bool)
        n621 = Select(t=i16 1, s=w1140, f=w1143) -> (s? t:f=w1142:i16)
        n622 = feedback-in #48(w1142) -> ()
        n623 = Divide(x=w1108, y=w1111) -> (x/y=w1107:fxp<+/-,16,1>)
        n624 = feedback #49(w1114) -> (w1112:bool)
        n625 = feedback #50(w1114) -> (w1130:bool)
        n626 = case shown="2" w1137 {
          tunnel: w1111 -> [w1168 w1175 _]
          tunnel: ["Set 1" "Set 2" "Set 3"] -> w1135
          tunnel: ["AI to FIFO" w1177 w1182] -> w1129
          tunnel: w1130 -> [_ w1177 w1182]
          tunnel: ["Trap Pos to FIFO" w1176 w1181] -> w1113
          tunnel: w1112 -> [_ w1176 w1181]
          tunnel: w1107 -> [w1167 w1174 _]
          tunnel: [w1166 w1172 FALSE] -> w1094
          tunnel: [w1165 w1173 u64 0 ("BD1 Frequency Out 2")] -> w1093
          frame 1, Default {
            n627 = local read "BD1 Frequency Out 1"() -> (w1165:u64)
            n628 = Compound Arithmetic op=AND("Trap Pos to FIFO", "Set 1", "AI to FIFO") -> (w1166:bool)
            "AI2 Y Sum Set 1" <- w1168
            "AI1 X Set 1" <- w1167
          }
          frame 2 {
            n629 = local read "BD1 Frequency Out 2"() -> (w1173:u64)
            n630 = Compound Arithmetic op=AND(w1176, "Set 2", w1177) -> (w1172:bool)
            "AI2 Y Sum Set 2" <- w1175
            "AI1 X Set 2" <- w1174
          }
          frame 3 {
          }
        }
        n631 = And(x=w1135, y=w1129) -> (x .and. y?=w1136:bool)
        n632 = case shown="True" w1136 {
          tunnel: w1145 -> [_ w1196]
          tunnel: w1110 -> [_ w1195]
          tunnel: w1111 -> [_ w1194]
          tunnel: w1144 -> [_ w1193]
          tunnel: w1134 -> [_ w1192]
          tunnel: w1133 -> [_ w1191]
          tunnel: w1132 -> [_ w1190]
          tunnel: w1131 -> [_ w1189]
          tunnel: 0 ("DMA buffer timeout") -> [_ w1198]
          frame False {
          }
          frame True {
            n633 = Build Array(w1196, w1195, w1194, w1193, w1192, w1191, w1190, w1189) -> (w1197:i16[])
            n634 = for {
              tunnel: w1197 -> [w1200] mode=indexing
              tunnel: w1198 -> [w1201]
              tunnel: [w1199] -> w1187 mode=indexing
              n635 = xnode ("FIFO Write")("Element"=w1200, "Timeout"=w1201) -> ("Timed Out?"=w1199:bool)  [unwired: 1 in, 1 out]
            }
            n636 = Or Array Elements(Boolean array=w1187) -> (logical OR=w1184:bool)
            n637 = Boolean To (0,1)(Boolean=w1184) -> (0, 1=w1186:i16)
            n638 = feedback #51(u16 0) -> (w1185:u16)
            n639 = Add(x=w1186, y=w1185) -> (x+y=w1183:u16)
            "Trap AI FIFO Timeout" <- w1183
            n640 = feedback-in #51(w1183) -> ()
          }
        }
        n641 = feedback-in #49(w1113) -> ()
        n642 = feedback-in #50(w1129) -> ()
        n643 = case shown="True" w1094 {
          tunnel: w1093 -> [_ w1151]
          tunnel: [u8 0 w1148] -> w1092
          frame False {
          }
          frame True {
            n644 = Split Number(x=w1151) -> (hi(x)=w1152:u32, lo(x)=w1153:u32)
            n645 = Split Number(x=w1152) -> (lo(x)=w1154:u16)  [unwired: 1 out]
            n646 = Split Number(x=w1153) -> (hi(x)=w1155:u16, lo(x)=w1156:u16)
            n647 = Build Array "BD 1 nu Stack"(w1154, w1155, w1156) -> (w1150:u16[])
            n648 = for {
              tunnel: w1150 -> [w1163] mode=indexing
              shift-right: [w1159] -> w1148
              shift-left: u8 0 -> [w1160]
              n649 = xnode ("FIFO Method Node")("Element"=w1163, "Timeout"="Trap FIFO Set Timeout") -> ("Timed Out?"=w1162:bool)  [unwired: 1 in, 1 out]
              n650 = Boolean To (0,1)(Boolean=w1162) -> (0, 1=w1161:i16)
              n651 = To Unsigned Byte Integer(number=w1161) -> (unsigned 8bit integer=w1158:u8)
              n652 = Add(x=w1158, y=w1160) -> (x+y=w1159:u8)
            }
          }
        }
        n653 = To Unsigned Word Integer(number=w1092) -> (unsigned 16bit integer=w1091:u16)
        n654 = feedback #52(u16 0) -> (w1105:u16)
        n655 = Add(x=w1091, y=w1105) -> (x+y=w1104:u16)
        "Trap Pos FIFO Timeout" <- w1104
        n656 = feedback-in #52(w1104) -> ()
        n657 = feedback-in #53(w1128) -> ()
        n658 = feedback #53(w1128) -> (w1127:u16)
        n659 = Subtract(x=w1128, y=w1127) -> (x-y=w1126:u16)
        n660 = xnode "FPGA I/O Node"("Connector1/DIO31"=FALSE ("Connector1/DIO34")) -> ()  [unwired: 1 in, 1 out]
        n661 = Subtract(x=w1126, y=w1125) -> (x-y=w1096:u16)
        n662 = Boolean To (0,1)(Boolean="+ phase") -> (0, 1=w1121:i16)
        n663 = Multiply(x=w1121, y="Phase count adjustment") -> (x*y=w1115:i16)
        n664 = Subtract(x="ai count", y=w1096) -> (x-y=w1119:u16)
        n665 = Number To Boolean Array(number=w1096) -> (Boolean array=w1097:bool[])
        n666 = feedback #54(i16 0) -> (w1117:i16)
        n667 = Add(x=w1119, y=w1115) -> (x+y=w1118:u16)
        n668 = Subtract(x=w1117, y=w1115) -> (x-y=w1116:i16)
        "Relative phase" <- w1116
        n669 = feedback-in #54(w1116) -> ()
        n670 = Or Array Elements(Boolean array=w1097) -> (logical OR=w1095:bool)
        n671 = Boolean To (0,1)(Boolean=w1095) -> (0, 1=w1102:i16)
        n672 = To Unsigned Byte Integer(number=w1102) -> (unsigned 8bit integer=w1099:u8)
        n673 = feedback #55(u8 0) -> (w1100:u8)
        n674 = Add(x=w1099, y=w1100) -> (x+y=w1098:u8)
        "AI Late Counter" <- w1098
        n675 = feedback-in #55(w1098) -> ()
      }
    }
  }
  n676 = node-c288(w8) -> ()
  n677 = while "APD 3 Counter" {
    tunnel: w2 -> [_]
    stop <- FALSE stop-if-true
    n678 = flat-sequence {
      frame #0 {
        n679 = xnode "FPGA I/O Method Node"("FPGA I/O In"=refnum<k21> "Connector0/DIO2" ("APD 2 DO"), "Timeout"=-1) -> ()  [unwired: 2 out]
      }
      frame #1 {
        n680 = local read "APD3 out state"() -> (w1205:bool)
        n681 = case shown="False" w1205 {
          frame False {
            n682 = local read "APD 3 Counts 0"() -> (w1207:u32)
            n683 = Increment(x=w1207) -> (x+1=→"APD 3 Counts 0":u32)
          }
          frame True {
            n684 = local read "APD 3 Counts 1"() -> (w1209:u32)
            n685 = Increment(x=w1209) -> (x+1=→"APD 3 Counts 1":u32)
          }
        }
      }
    }
  }
  n686 = while "APD 3 Gating" {
    shift-right: [w1213] -> _
    shift-left: w2 -> [w1218]
    shift-right: [w1212] -> _
    shift-left: w6 -> [w1210]
    stop <- FALSE stop-if-true
    n687 = flat-sequence {
      tunnel: w1218 -> [w1221]
      tunnel: [w1222] -> w1216
      tunnel: [w1221] -> w1214
      tunnel: [w1220] -> w1211
      tunnel: w1210 -> [w1220]
      tunnel: [w1225] -> w1217
      tunnel: w1216 -> [w1225]
      tunnel: [w1224] -> w1215
      tunnel: w1214 -> [w1224]
      tunnel: w1211 -> [w1223]
      tunnel: [w1242] -> w1213
      tunnel: w1217 -> [w1254]
      tunnel: w1215 -> [w1251]
      tunnel: [w1246] -> w1212
      frame #0 {
        n688 = call "Loop Timer15"("Count(Ticks)"=w1221) -> ("Tick Count(Ticks)"=w1222:u16)
      }
      frame #1 {
        # "Signal is then sent through \na transistor before APD"
        n689 = xnode "FPGA I/O Node"("Connector0/DIO9"=w1223) -> ()  [unwired: 1 in, 1 out]
      }
      frame #2 {
        n690 = local read "APD Gate OFF Count"() -> (w1227:u16)
        n691 = local read "APD Gate ON Count"() -> (w1228:u16)
        n692 = feedback #56(TRUE) -> (w1248:bool)
        n693 = feedback-in #57(w1254) -> ()
        n694 = feedback #57(w1254) -> (w1253:u16)
        n695 = Not(x=w1248) -> (.not. x?=w1245:bool)
        n696 = feedback-in #56(w1245) -> ()
        n697 = Subtract(x=w1254, y=w1253) -> (x-y=w1252:u16)
        n698 = Select(t=w1228, s=w1245, f=w1227) -> (s? t:f=w1250:u16)
        n699 = Subtract(x=w1252, y=w1251) -> (x-y=w1230:u16)
        n700 = Subtract(x=w1250, y=w1230) -> (x-y=w1241:u16)
        n701 = Number To Boolean Array(number=w1230) -> (Boolean array=w1231:bool[])
        n702 = Or Array Elements(Boolean array=w1231) -> (logical OR=w1229:bool)
        n703 = Boolean To (0,1)(Boolean=w1229) -> (0, 1=w1236:i16)
        n704 = Boolean To (0,1)(Boolean="+ phase (APD 3 Gate)") -> (0, 1=w1239:i16)
        n705 = To Unsigned Byte Integer(number=w1236) -> (unsigned 8bit integer=w1233:u8)
        n706 = Multiply(x=w1239, y="Phase count adjustment (APD 3 Gate)") -> (x*y=w1237:i16)
        n707 = feedback #58(u8 0) -> (w1234:u8)
        n708 = Add(x=w1233, y=w1234) -> (x+y=w1232:u8)
        "APD 3 Gate Late Counter" <- w1232
        n709 = feedback-in #58(w1232) -> ()
        n710 = Add(x=w1241, y=w1237) -> (x+y=w1242:u16)
        n711 = feedback #59(i16 0) -> (w1244:i16)
        n712 = Subtract(x=w1244, y=w1237) -> (x-y=w1243:i16)
        "APD 3 Gate Relative Phase" <- w1243
        n713 = feedback-in #59(w1243) -> ()
        n714 = local read "APD Gate Operating Mode"() -> (w1226:u8)
        n715 = case shown="2" w1226 {
          tunnel: [TRUE FALSE w1260] -> w1246
          tunnel: w1248 -> [_ _ w1258]
          frame 0, Default {
          }
          frame 1 {
          }
          frame 2 {
            n716 = local read "Invert APD Gate"() -> (w1257:bool)
            n717 = Not(x=w1258) -> (.not. x?=w1259:bool)
            n718 = Select(t=w1259, s=w1257, f=w1258) -> (s? t:f=w1260:bool)
          }
        }
      }
    }
  }
  n719 = while "633 nm red  fluorescent laser interlacing (DO to IA 633 nm AOM ME amp)." {
    shift-right: [w1264] -> _
    shift-left: w2 -> [w1269]
    shift-right: [w1263] -> _
    shift-left: w3 -> [w1261]
    stop <- FALSE stop-if-true
    n720 = flat-sequence {
      tunnel: w1269 -> [w1272]
      tunnel: [w1273] -> w1267
      tunnel: [w1272] -> w1265
      tunnel: [w1271] -> w1262
      tunnel: w1261 -> [w1271]
      tunnel: [w1276] -> w1268
      tunnel: w1267 -> [w1276]
      tunnel: [w1275] -> w1266
      tunnel: w1265 -> [w1275]
      tunnel: w1262 -> [w1274]
      tunnel: [w1285] -> w1264
      tunnel: w1268 -> [w1305]
      tunnel: w1266 -> [w1302]
      tunnel: [w1294] -> w1263
      frame #0 {
        n721 = call "Loop Timer11"("Count(Ticks)"=w1272) -> ("Tick Count(Ticks)"=w1273:u16)
      }
      frame #1 {
        # "Then to PRL 440 amp"
        n722 = xnode "FPGA I/O Node"("Connector1/DIO32"=w1274) -> ()  [unwired: 1 in, 1 out]
      }
      frame #2 {
        n723 = feedback-in #60(w1305) -> ()
        n724 = feedback #60(w1305) -> (w1304:u16)
        n725 = Subtract(x=w1305, y=w1304) -> (x-y=w1303:u16)
        n726 = Subtract(x=w1303, y=w1302) -> (x-y=w1278:u16)
        n727 = Number To Boolean Array(number=w1278) -> (Boolean array=w1279:bool[])
        n728 = Or Array Elements(Boolean array=w1279) -> (logical OR=w1277:bool)
        n729 = Boolean To (0,1)(Boolean="+ phase (RI)") -> (0, 1=w1290:i16)
        n730 = Multiply(x=w1290, y="Phase count adjustment (RI)") -> (x*y=w1287:i16)
        n731 = Boolean To (0,1)(Boolean=w1277) -> (0, 1=w1284:i16)
        n732 = To Unsigned Byte Integer(number=w1284) -> (unsigned 8bit integer=w1281:u8)
        n733 = feedback #61(i16 0) -> (w1288:i16)
        n734 = feedback #62(u8 0) -> (w1282:u8)
        n735 = Add(x=w1281, y=w1282) -> (x+y=w1280:u8)
        "RI Late Counter" <- w1280
        n736 = feedback-in #62(w1280) -> ()
        n737 = Subtract(x=w1288, y=w1287) -> (x-y=w1286:i16)
        "RI Relative phase" <- w1286
        n738 = feedback-in #61(w1286) -> ()
        n739 = feedback #63(TRUE) -> (w1297:bool)
        n740 = case shown="2" "Red Laser Operating Mode" {
          tunnel: [TRUE FALSE w1311] -> w1294
          tunnel: w1297 -> [_ _ w1308]
          frame 0, Default {
          }
          frame 1 {
          }
          frame 2 {
            n741 = Not(x=w1308) -> (.not. x?=w1310:bool)
            n742 = Select(t=w1310, s="Invert RI", f=w1308) -> (s? t:f=w1311:bool)
          }
        }
        n743 = Not(x=w1297) -> (.not. x?=w1293:bool)
        n744 = Select(t="Red interlace ON count", s=w1293, f="Red interlace OFF count") -> (s? t:f=w1299:u16)
        n745 = Subtract(x=w1299, y=w1278) -> (x-y=w1291:u16)
        n746 = Add(x=w1291, y=w1287) -> (x+y=w1285:u16)
        n747 = feedback-in #63(w1293) -> ()
      }
    }
  }
  n748 = while "473 nm blue  fluorescent laser interlacing (DO to blue laser digital control input)." {
    shift-right: [w1315] -> _
    shift-left: w2 -> [w1320]
    shift-right: [w1314] -> _
    shift-left: w3 -> [w1312]
    stop <- FALSE stop-if-true
    n749 = flat-sequence {
      tunnel: w1320 -> [w1323]
      tunnel: [w1324] -> w1318
      tunnel: [w1323] -> w1316
      tunnel: [w1322] -> w1313
      tunnel: w1312 -> [w1322]
      tunnel: [w1327] -> w1319
      tunnel: w1318 -> [w1327]
      tunnel: [w1326] -> w1317
      tunnel: w1316 -> [w1326]
      tunnel: w1313 -> [w1325]
      tunnel: [w1336] -> w1315
      tunnel: w1319 -> [w1356]
      tunnel: w1317 -> [w1353]
      tunnel: [w1345] -> w1314
      frame #0 {
        n750 = call "Loop Timer14"("Count(Ticks)"=w1323) -> ("Tick Count(Ticks)"=w1324:u16)
      }
      frame #1 {
        n751 = xnode "FPGA I/O Node"("Connector1/DIO28"=w1325) -> ()  [unwired: 1 in, 1 out]
      }
      frame #2 {
        n752 = feedback-in #64(w1356) -> ()
        n753 = feedback #64(w1356) -> (w1355:u16)
        n754 = Subtract(x=w1356, y=w1355) -> (x-y=w1354:u16)
        n755 = Subtract(x=w1354, y=w1353) -> (x-y=w1329:u16)
        n756 = Number To Boolean Array(number=w1329) -> (Boolean array=w1330:bool[])
        n757 = Or Array Elements(Boolean array=w1330) -> (logical OR=w1328:bool)
        n758 = Boolean To (0,1)(Boolean="+ phase (BI D)") -> (0, 1=w1341:i16)
        n759 = Multiply(x=w1341, y="Phase count adjustment (BI D)") -> (x*y=w1338:i16)
        n760 = Boolean To (0,1)(Boolean=w1328) -> (0, 1=w1335:i16)
        n761 = To Unsigned Byte Integer(number=w1335) -> (unsigned 8bit integer=w1332:u8)
        n762 = feedback #65(i16 0) -> (w1339:i16)
        n763 = feedback #66(u8 0) -> (w1333:u8)
        n764 = Add(x=w1332, y=w1333) -> (x+y=w1331:u8)
        "Blue Late Counter (D)" <- w1331
        n765 = feedback-in #66(w1331) -> ()
        n766 = Subtract(x=w1339, y=w1338) -> (x-y=w1337:i16)
        "BI Relative phase (D)" <- w1337
        n767 = feedback-in #65(w1337) -> ()
        n768 = feedback #67(TRUE) -> (w1348:bool)
        n769 = case shown="2" "Blue Laser Operating Mode (D)" {
          tunnel: [TRUE FALSE w1362] -> w1345
          tunnel: w1348 -> [_ _ w1359]
          frame 0, Default {
          }
          frame 1 {
          }
          frame 2 {
            n770 = Not(x=w1359) -> (.not. x?=w1361:bool)
            n771 = Select(t=w1361, s="Invert BI (D)", f=w1359) -> (s? t:f=w1362:bool)
          }
        }
        n772 = Not(x=w1348) -> (.not. x?=w1344:bool)
        n773 = Select(t="Blue interlace ON count (D)", s=w1344, f="Blue interlace OFF count (D)") -> (s? t:f=w1350:u16)
        n774 = Subtract(x=w1350, y=w1329) -> (x-y=w1342:u16)
        n775 = Add(x=w1342, y=w1338) -> (x+y=w1336:u16)
        n776 = feedback-in #67(w1344) -> ()
      }
    }
  }
  n777 = while "Blue fluorescent laser interlacing (AO control direct to laser)." {
    shift-right: [w1368] -> _
    shift-left: w2 -> [w1371]
    shift-right: [w1365] -> _
    shift-left: i16 0 -> [w1363]
    stop <- FALSE stop-if-true
    n778 = flat-sequence {
      tunnel: w1371 -> [w1374]
      tunnel: [w1375] -> w1370
      tunnel: [w1374] -> w1369
      tunnel: [w1373] -> w1364
      tunnel: w1363 -> [w1373]
      tunnel: [w1378] -> w1367
      tunnel: w1370 -> [w1378]
      tunnel: [w1377] -> w1366
      tunnel: w1369 -> [w1377]
      tunnel: w1364 -> [w1376]
      tunnel: [w1388] -> w1368
      tunnel: [w1404] -> w1365
      tunnel: w1367 -> [w1416]
      tunnel: w1366 -> [w1413]
      frame #0 {
        n779 = call "Loop Timer13"("Count(Ticks)"=w1374) -> ("Tick Count(Ticks)"=w1375:u16)
      }
      frame #1 {
        n780 = xnode "FPGA I/O Node"("Connector0/AO3"=w1376) -> ()  [unwired: 1 in, 1 out]
      }
      frame #2 {
        n781 = Subtract(x="Blue OFF count (AO)", y="Blue current ON count adj (AO)") -> (x-y=w1397:u16)
        n782 = feedback-in #68(w1416) -> ()
        n783 = feedback #68(w1416) -> (w1415:u16)
        n784 = Add(x="Blue current ON count adj (AO)", y="Blue ON count (AO)") -> (x+y=w1398:u16)
        n785 = Subtract(x=w1416, y=w1415) -> (x-y=w1414:u16)
        n786 = Subtract(x=w1414, y=w1413) -> (x-y=w1381:u16)
        n787 = Number To Boolean Array(number=w1381) -> (Boolean array=w1382:bool[])
        n788 = Boolean To (0,1)(Boolean="+ phase (BI AO)") -> (0, 1=w1394:i16)
        n789 = Or Array Elements(Boolean array=w1382) -> (logical OR=w1380:bool)
        n790 = Boolean To (0,1)(Boolean=w1380) -> (0, 1=w1387:i16)
        n791 = Multiply(x=w1394, y="Phase count adjustment (BI AO)") -> (x*y=w1390:i16)
        n792 = To Unsigned Byte Integer(number=w1387) -> (unsigned 8bit integer=w1383:u8)
        n793 = feedback #69(u8 0) -> (w1385:u8)
        n794 = Add(x=w1383, y=w1385) -> (x+y=w1384:u8)
        "BI Late Counter (AO)" <- w1384
        n795 = feedback-in #69(w1384) -> ()
        n796 = feedback #70(i16 0) -> (w1391:i16)
        n797 = Subtract(x=w1391, y=w1390) -> (x-y=w1389:i16)
        "BI Relative phase (AO)" <- w1389
        n798 = feedback-in #70(w1389) -> ()
        n799 = feedback #71(TRUE) -> (w1408:bool)
        n800 = case shown="2" "BI Operating Mode (AO)" {
          tunnel: [TRUE FALSE w1432] -> w1399
          tunnel: w1408 -> [_ _ w1429]
          frame 0, Default {
          }
          frame 1 {
          }
          frame 2 {
            n801 = Not(x=w1429) -> (.not. x?=w1431:bool)
            n802 = Select(t=w1431, s="Invert BI (AO)", f=w1429) -> (s? t:f=w1432:bool)
          }
        }
        n803 = And(x=w1399, y="Blue FB On/Off") -> (x .and. y?=w1400:bool)
        n804 = case shown="True" w1400 {
          tunnel: "BI Current Out" -> [w1417 _]
          tunnel: [w1417 w1419] -> w1403
          frame False {
          }
          frame True {
            n805 = local read "Blue Intensity"() -> (w1418:i16)
            n806 = Bundle("P5"="P5", "I5"="I5", "D5"="D5") -> (w1420:cluster{"P5":i16, "I5":i16, "D5":i16})  [unwired: 1 in]
            n807 = call "Slower PID.vi"("process variable"=w1418, "reset?"="Blue FB Reset", "setpoint"="Blue FB Setpoint", "PID gains (x 2^8)"=w1420, "output range"=cluster{"output high":i16, "output low":i16} {"output high"=32767, "output low"=0} ("Green FB output range")) -> ("output"=w1419:i16)  [unwired: 10 out]
          }
        }
        n808 = Not(x=w1408) -> (.not. x?=w1405:bool)
        n809 = Select(t=w1398, s=w1405, f=w1397) -> (s? t:f=w1410:u16)
        n810 = Subtract(x=w1410, y=w1381) -> (x-y=w1392:u16)
        n811 = Add(x=w1392, y=w1390) -> (x+y=w1388:u16)
        n812 = feedback-in #71(w1405) -> ()
        n813 = Boolean To (0,1)(Boolean=w1399) -> (0, 1=w1379:i16)
        n814 = Multiply(x=w1379, y=w1403) -> (x*y=w1404:i16)
      }
    }
  }
